vi "Marvin.vi"() -> ()   [LabVIEW 2017]
uses:
  Marvin ATP Remake 1.5.18/PCAN_Driver/ControlCAN.llb/CAN Channel.ctl
  Marvin ATP Remake 6.5.18 - Copy/PCAN_Driver/ControlCAN.llb/DevType.ctl
  Marvin ATP Remake 30.5.18/PCAN_Driver/ControlCAN.llb/VCI_INIT_CONFIG.ctl
  Marvin ATP Remake 30.5.18/PCAN_Driver/ControlCAN.llb/InitFlag.ctl
  Marvin ATP Remake 6.5.18/PCAN_Driver/ControlCAN.llb/Fliter.ctl
  Marvin ATP Remake 6.5.18/PCAN_Driver/ControlCAN.llb/Mode.ctl
  <vilib>/Utility/miscctls.llb/LVMinMaxIncTypeDef.ctl
  PCAN_Driver/ControlCAN.llb/VCI_CAN_OBJ.ctl
  Marvin ATP Remake 30.5.18/PCAN_Driver/ControlCAN.lvlib
panel:
  in  "Graph Plot":bool
  in  "Get":bool
  in  "Set":bool
  out "Array 2":dbl[](array[numeric])
  in  "Clear Data Array":bool
  in  "PlayPause Data Array":bool
  out "CAN Data":cluster{"Frame Data":u64, "Frame ID":u32}[](array[cluster]) {"Frame ID" format="%.0x"; "Frame Data" format="%016x"}
  out "Waveform Chart":dbl(graph)
  in  "Help Button":bool
  in  "Clear Monitor":bool
  out "Array":u64[][](array[numeric]) format="%016x"
  out "Ambient Over temp":bool
  out "Ambient Sensor temp":bool
  out "Ambient Temperature":dbl
  in  "Motor Over Temp":bool
  in  "Speed control":bool
  out "Unit Adress":string
  in  "Serial Send":bool
  in  "Index":u16(ring) items=["1"=1, "2"=2, "3"=3]
  out "read buffer":string
  in  "SetGet":enum16{"Get", "Set"}(ring)
  in  "Function":T1(ring)
  in  "Value":dbl
  in  "Value 1/2":enum16{"1", "2"}(ring)
  out "Msg Count":u32
  in  "Param to Set":u16(ring) items=["EBAY 5F"=95, "AHU 3F"=63, "AHU 2F"=47]
  out "UUT":u8
  out "Horizontal Progress Bar":i32(slide) min=0 max=48 scale=0.0..50.0
  in  "Set Param.":bool
  in  "Serial Monitor":bool caption="Graph Button"
  in  "Serial Com":bool
  in  "VISA resource name":refnum<visa-resource-name>="COM6"
  out "Serial Status":bool
  in  "Graph Button":bool
  in  "Refresh Button":bool
  out "Data Send":u64 format="%016x"
  in  "Motor Speed RPM":u16
  out "Under voltage/Over voltage":bool
  out "Speed error":bool
  out "Derated drive temp":bool
  out "Motor Over temperature":bool
  out "Commutation err":bool
  out "Motor Sensor temp Fauilre":bool
  out "Drive Over temperature":bool
  out "Drive Sensor temp Failure":bool
  out "Motor Phase Current RMS":dbl
  out "ECS State":u16
  out "Motor Speed RPM":dbl
  out "Motor Stator Temp.":dbl
  out "Power transistor Heat sink Temp.":dbl
  out "Phase Current":dbl
  out "DC Voltage":dbl
  in  "Can Send":bool
  in  "Stop":bool
  out "Config_CANAT":T8 {"DevType" items=["USB-CAN"=3, "USB-CAN2"=4]; "CanIndex" items=["通道1", "通道2"]; "VCI_INIT_CONFIG"."Fliter" items=["接收所有类型"=3, "只接收标准帧"=4, "只接收扩展帧"=7]; "VCI_INIT_CONFIG"."Mode" items=["正常工作", "自测模式（环回）", "仅侦听模式"]; "VCI_INIT_CONFIG"."InitFlag" items=["使用Flash参数", "使用界面设置参数"]}
  in  "Channel 2":T3 caption="Channel" items=["Channel 1", "Channel 2"]
  out "CAN Status":bool
  out "Driver Version":string
  out "Hall Sensor Fault":bool
  out "Motor Phase Current":dbl
  in  "Motor Phase Current":u16
  # "ver 0.0.b"
  # "Redler"
  # "REDLER TECHNOLOGIES LTD"
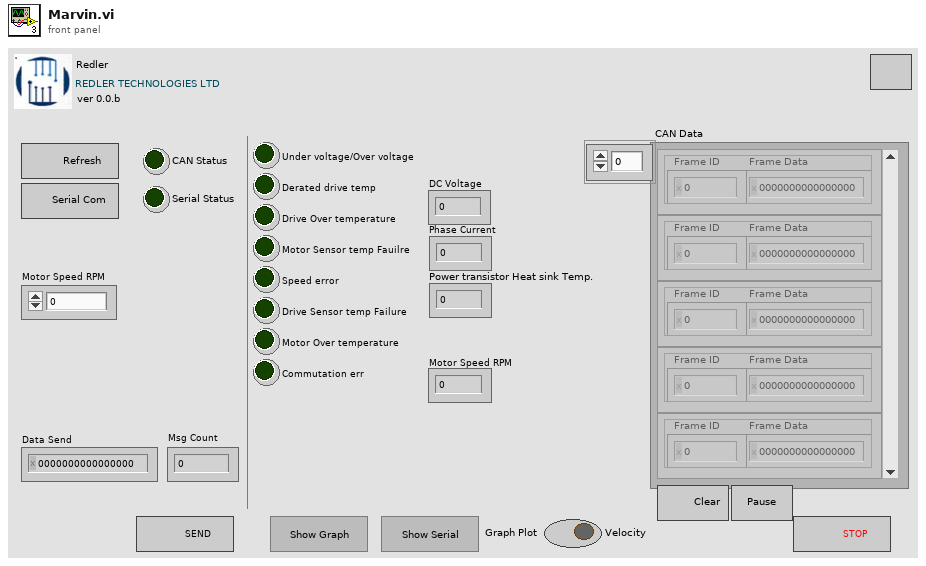
[diagram p1: front panel]
types:
  T1 = enum16{"Enable Conf. EP=1", "Serial Number", "Temperature", "Unit Adress", "Calibration", "Velocity", "Version"}
  T2 = typedef "ControlCAN.lvlib/DevType.ctl" = u32
  T3 = typedef "ControlCAN.lvlib/CAN Channel.ctl" = u32
  T4 = typedef "ControlCAN.lvlib/VCI_INIT_CONFIG.ctl" = cluster{"AccCode":u32, "AccMask":u32, "InitFlag":T5, "Fliter":T6, "Timing0":u8, "Timing1":u8, "Mode":T7}
  T5 = typedef "ControlCAN.lvlib/InitFlag.ctl" = u32
  T6 = typedef "ControlCAN.lvlib/Fliter.ctl" = u8
  T7 = typedef "ControlCAN.lvlib/Mode.ctl" = u8
  T8 = cluster{"DevType":T2, "DevIndex":u32, "CanIndex":T3, "VCI_INIT_CONFIG":T4}
  T9 = cluster{"ID":u32, "MSGTYPE":u8, "LEN":u8, "aDATA":u8[]}[]
  T10 = cluster{"ID":u32, "MSGTYPE":u8, "LEN":u8, "aDATA":u8[]}
  T11 = enum8{"Enabled", "Disabled", "Disabled and Grayed Out"}
  T12 = typedef "LVMinMaxIncTypeDef.ctl" = cluster{"Minimum":dbl, "Maximum":dbl, "Increment":dbl}
  T13 = enum32{"Invalid", "Standard", "Closed", "Hidden", "Minimized", "Maximized"}
  T14 = typedef "ControlCAN.lvlib/VCI_CAN_OBJ.ctl" = cluster{"ID":u32, "TimeStamp":u32, "TimeFlag":u8, "SendType":u8, "RemoteFlag":u8, "ExternFlag":u8, "DataLen":u8, "Data":u8[], "Reserved":u8[]}
  T15 = cluster{"Type":enum16{"接收", "发送"}, "Channel":T3, "Time":timestamp, "VCI_CAN_OBJ":T14}[]
  T16 = cluster{"Type":enum16{"接收", "发送"}, "Channel":T3, "Time":timestamp, "VCI_CAN_OBJ":T14}
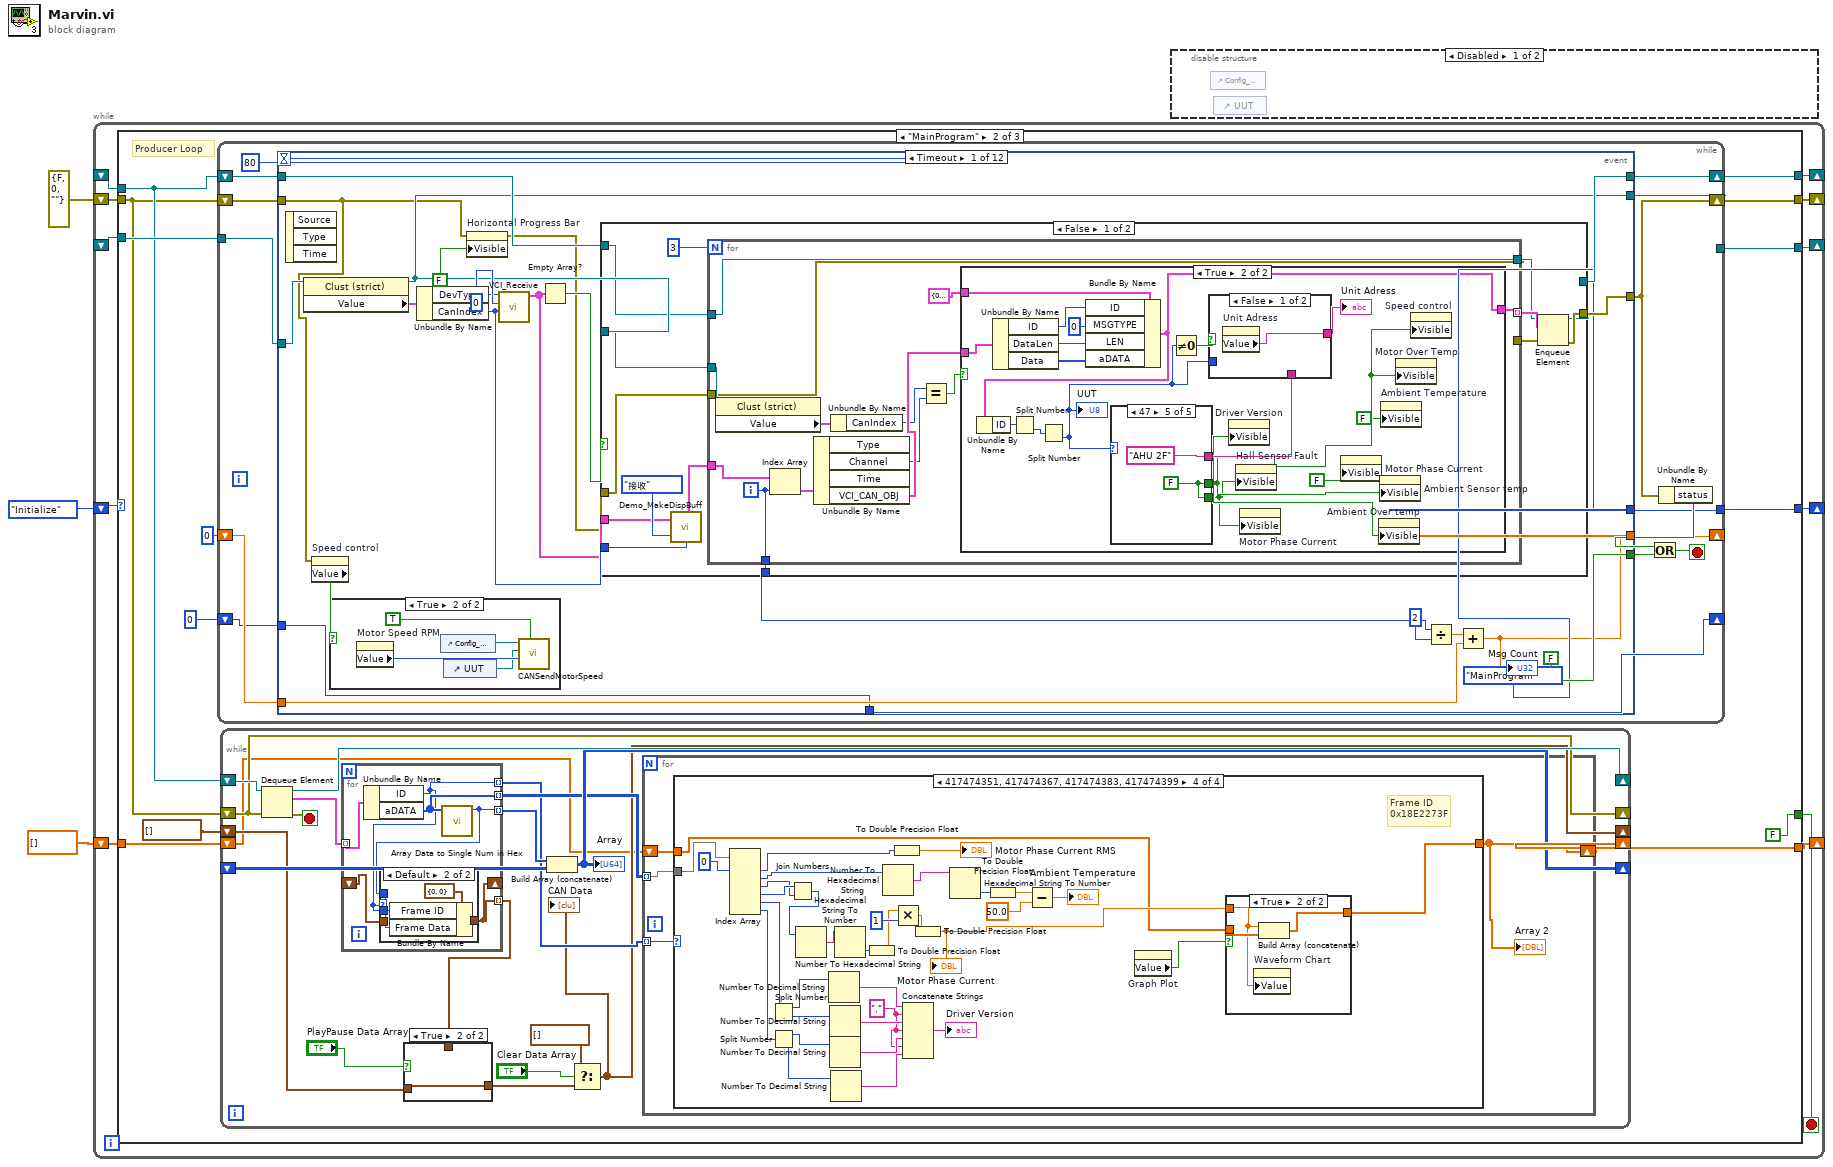
[diagram p0: block diagram]
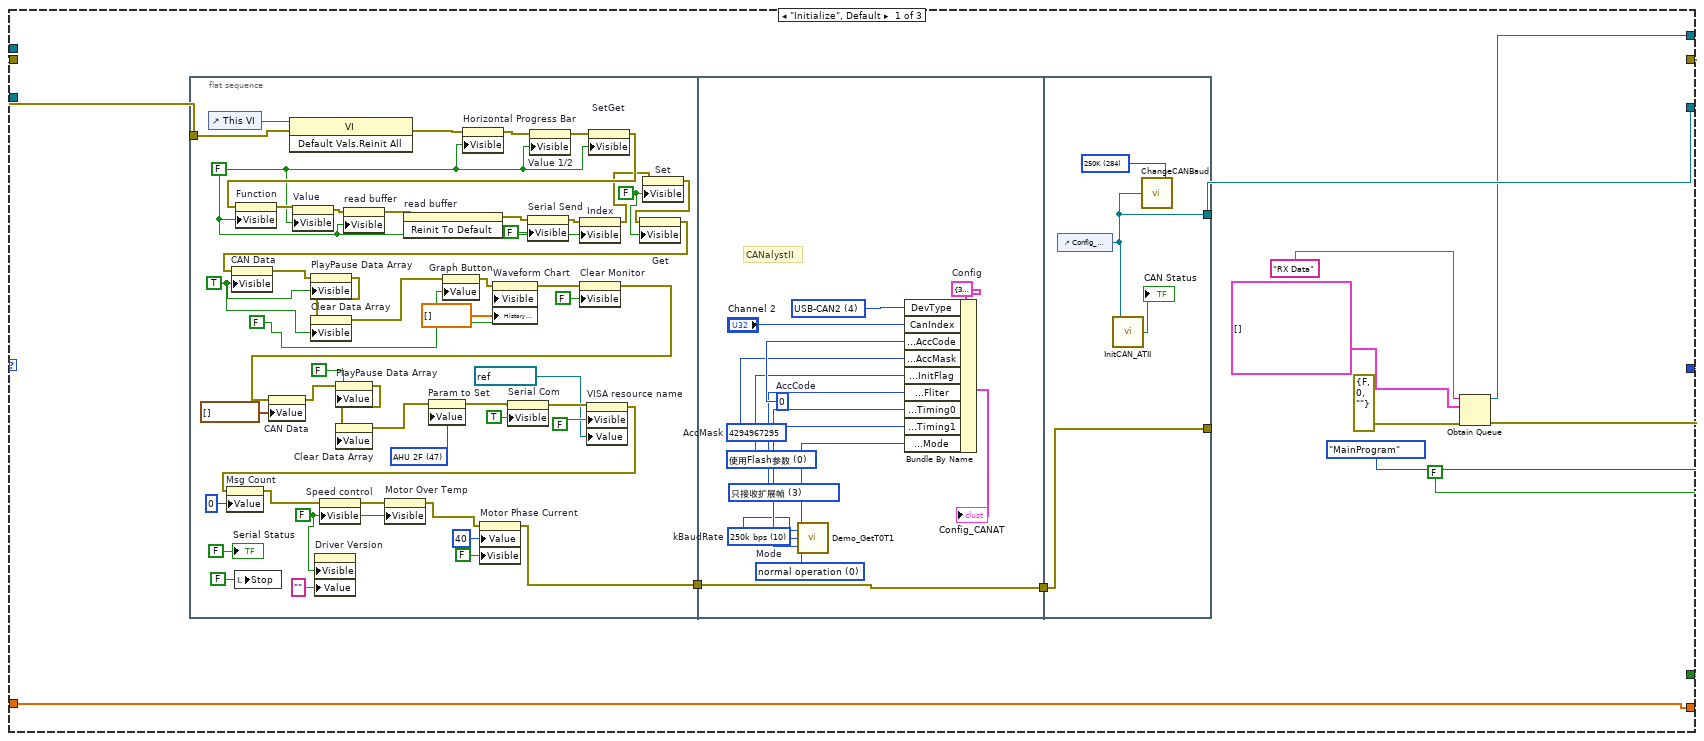
[diagram p3: hidden frame]
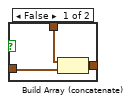
[diagram p4: hidden frame]
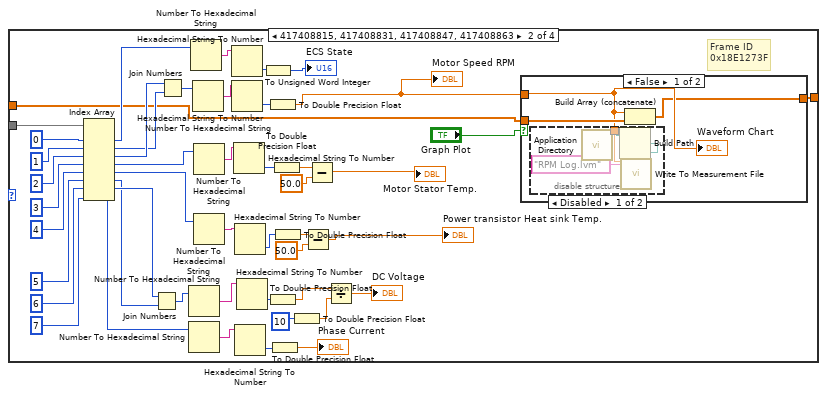
[diagram p6: hidden frame]
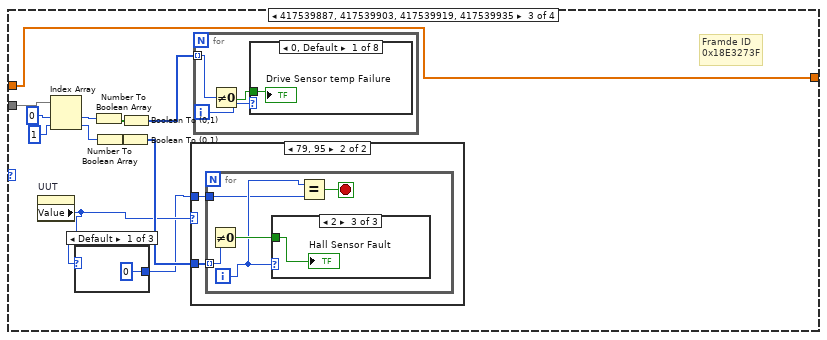
[diagram p9: hidden frame]
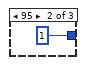
[diagram p10: hidden frame]
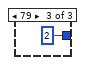
[diagram p11: hidden frame]
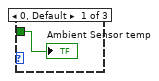
[diagram p13: hidden frame]
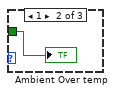
[diagram p14: hidden frame]
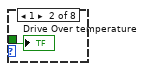
[diagram p15: hidden frame]
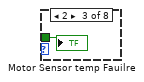
[diagram p16: hidden frame]
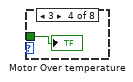
[diagram p17: hidden frame]
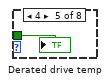
[diagram p18: hidden frame]
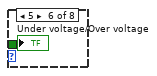
[diagram p19: hidden frame]
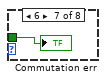
[diagram p20: hidden frame]
diagram:
  n1 = while {
    shift-right: [w9] -> _
    shift-left: enum16{"Stop", "MainProgram", "Initialize"}."Initialize" -> [w14]
    shift-right: [w13] -> _
    shift-left: _ -> [w12]
    shift-right: [w11] -> _
    shift-left: _ -> [w8]
    shift-right: [w10] -> _
    shift-left: errorcluster {"status"=FALSE, "code"=0, "source"=""} ("error out") -> [w7]
    shift-right: [w4] -> _
    shift-left: dbl[] [] -> [w5]
    stop <- w6 stop-if-true
    n2 = case shown="\"MainProgram\"" w14 {
      tunnel: [w26 w103 w1077] -> w13
      tunnel: w12 -> [_ w106 w1077]
      tunnel: [w22 w105 w1078] -> w11
      tunnel: [w21 w104 w1079] -> w10
      tunnel: [enum16{"Stop", "MainProgram", "Initialize"}."MainProgram" w102 enum16{"Stop", "MainProgram", "Initialize"}."Stop"] -> w9
      tunnel: w8 -> [_ w101 w1078]
      tunnel: w7 -> [w19 w100 w1080]
      tunnel: [FALSE ("Stop") FALSE ("Stop") w1076] -> w6
      tunnel: w5 -> [w15 w97 w1074]
      tunnel: [w15 w96 w1074] -> w4
      frame "Initialize", Default {
        n3 = flat-sequence {
          tunnel: w19 -> [w58]
          tunnel: [w34] -> w17
          tunnel: [w77] -> w18
          tunnel: w17 -> [w77]
          tunnel: [w91] -> w26
          tunnel: w18 -> [w90]
          tunnel: [w90] -> _
          frame #0 {
            w31 = FALSE ("Visible")
            w43 = FALSE ("PlayPause Data Array")
            w37 = FALSE ("Visible")
            w68 = u16 47 items=["EBAY 5F"=95, "AHU 3F"=63, "AHU 2F"=47] ("Param to Set")
            w38 = TRUE ("Visible")
            w52 = FALSE ("Visible")
            w42 = FALSE ("Graph Button")
            n4 = control-ref of="This VI"() -> (w76:refnum<vi>)
            n5 = local write "Stop"(FALSE ("Stop")) -> ()
            n6 = invoke class="VI" method="Default Vals.Reinit All"(reference=w76, error in=w58) -> (error out=w57:errorcluster)  [unwired: 1 in, 2 out]
            n7 = property on="Driver Version" class="Str"("Visible"=w37, "Value"="" ("Driver Version")) -> ()  [unwired: 2 in, 2 out]
            n8 = property on="Horizontal Progress Bar" class="Slide (strict)"(error in=w57, "Visible"=w52) -> (error out=w66:errorcluster)  [unwired: 1 in, 1 out]
            n9 = property on="Value 1/2" class="Enum (strict)"(error in=w66, "Visible"=w52) -> (error out=w65:errorcluster)  [unwired: 1 in, 1 out]
            n10 = property on="SetGet" class="Enum (strict)"(error in=w65, "Visible"=w52) -> (error out=w64:errorcluster)  [unwired: 1 in, 1 out]
            n11 = property on="Function" class="Enum (strict)"(error in=w64, "Visible"=w52) -> (error out=w63:errorcluster)  [unwired: 1 in, 1 out]
            n12 = property on="Value" class="DigNum (strict)"(error in=w63, "Visible"=w52) -> (error out=w62:errorcluster)  [unwired: 1 in, 1 out]
            n13 = property on="read buffer" class="Str"(error in=w62, "Visible"=w52) -> (error out=w54:errorcluster)  [unwired: 1 in, 1 out]
            n14 = invoke on="read buffer" class="Str" method="Reinit To Default"(error in=w54) -> (error out=w53:errorcluster)  [unwired: 2 in, 2 out]
            n15 = property on="Serial Send" class="Bool (strict)"(error in=w53, "Visible"=FALSE) -> (error out=w61:errorcluster)  [unwired: 1 in, 1 out]
            n16 = property on="Index" class="Ring (strict)"(error in=w61, "Visible"=w52) -> (error out=w29:errorcluster)  [unwired: 1 in, 1 out]
            n17 = property on="Set" class="Bool (strict)"(error in=w29, "Visible"=w31) -> (error out=w30:errorcluster)  [unwired: 1 in, 1 out]
            n18 = property on="Get" class="Bool (strict)"(error in=w30, "Visible"=w31) -> (error out=w28:errorcluster)  [unwired: 1 in, 1 out]
            n19 = property on="CAN Data" class="Arr (strict)"(error in=w28, "Visible"=w38) -> (error out=w41:errorcluster)  [unwired: 1 in, 1 out]
            n20 = property on="PlayPause Data Array" class="Bool (strict)"(error in=w41, "Visible"=w38) -> (error out=w40:errorcluster)  [unwired: 1 in, 1 out]
            n21 = property on="Clear Data Array" class="Bool (strict)"(error in=w40, "Visible"=w38) -> (error out=w39:errorcluster)  [unwired: 1 in, 1 out]
            n22 = property on="Graph Button" class="Bool (strict)"(error in=w39, "Value"=w42) -> (error out=w50:errorcluster)  [unwired: 1 in, 1 out]
            n23 = property on="Waveform Chart" class="WFChart (strict)"(error in=w50, "Visible"=w42, "History Data"=dbl[] [] ("Waveform Chart")) -> (error out=w49:errorcluster)  [unwired: 1 in, 1 out]
            n24 = property on="Clear Monitor" class="Bool"(error in=w49, "Visible"=FALSE) -> (error out=w48:errorcluster)  [unwired: 1 in, 1 out]
            n25 = property on="CAN Data" class="Arr (strict)"(error in=w48, "Value"=cluster{"Frame Data":u64, "Frame ID":u32}[] [] ("CAN Data")) -> (error out=w46:errorcluster)  [unwired: 1 in, 1 out]
            n26 = property on="PlayPause Data Array" class="Bool (strict)"(error in=w46, "Value"=w43) -> (error out=w45:errorcluster)  [unwired: 1 in, 1 out]
            n27 = property on="Clear Data Array" class="Bool (strict)"(error in=w45, "Value"=w43) -> (error out=w44:errorcluster)  [unwired: 1 in, 1 out]
            n28 = property on="Param to Set" class="Ring (strict)"(error in=w44, "Value"=w68) -> (error out=w60:errorcluster)  [unwired: 1 in, 1 out]
            n29 = property on="Serial Com" class="Bool"(error in=w60, "Visible"=TRUE) -> (error out=w73:errorcluster)  [unwired: 1 in, 1 out]
            n30 = property on="VISA resource name" class="VISAName"(error in=w73, "Visible"=FALSE, "Value"=refnum<visa-resource-name> "COM1" ("VISA resource name")) -> (error out=w59:errorcluster)  [unwired: 1 in, 1 out]
            n31 = property on="Msg Count" class="DigNum (strict)"(error in=w59, "Value"=u32 0 ("Msg Count")) -> (error out=w56:errorcluster)  [unwired: 1 in, 1 out]
            n32 = property on="Speed control" class="Bool (strict)"(error in=w56, "Visible"=w37) -> (error out=w55:errorcluster)  [unwired: 1 in, 1 out]
            n33 = property on="Motor Over Temp" class="Bool (strict)"(error in=w55, "Visible"=w37) -> (error out=w35:errorcluster)  [unwired: 1 in, 1 out]
            n34 = property on="Motor Phase Current" class="DigNum (strict)"(error in=w35, "Value"=u16 40 ("Motor Phase Current"), "Visible"=FALSE) -> (error out=w34:errorcluster)  [unwired: 1 in, 1 out]
            "Serial Status" <- FALSE ("Serial Status")
          }
          frame #1 {
            w81 = u32 4294967295  # AccMask
            w80 = T5 0 items=["使用Flash参数", "使用界面设置参数"] ("InitFlag")
            w78 = T7 0 items=["normal operation", "Listen-only mode", "test mode"]  # Mode
            w79 = T6 3 items=["接收所有类型"=1, "只接收标准帧"=2, "只接收扩展帧"=3] ("Fliter")
            w85 = u8 10 items=["5k bps"=1, "10k bps"=2, "20k bps"=3, "40k bps"=4, "50k bps"=5, "80k bps"=6, "100k bps"=7, "125k bps"=8, "200k bps"=9, "250k bps"=10, "400k bps"=11, "500k bps"=12, "666k bps"=13, "800k bps"=14, "1000k bps"=15, "33.33k bps"=16, "66.66k bps"=17, "83.33k bps"=18]  # kBaudRate
            w82 = u32 0  # AccCode
            w83 = T2 4 items=["USB-CAN"=3, "USB-CAN2"=4] ("DevType")
            w84 = T8 {"DevType"=3, "DevIndex"=0, "CanIndex"=0, "VCI_INIT_CONFIG"={"AccCode"=0, "AccMask"=0, "InitFlag"=1, "Fliter"=7, "Timing0"=0, "Timing1"=0, "Mode"=0}}  # Config
            # "CANalystII"
            n35 = call "Demo_GetT0T1.vi"("kBaudRate"=w85) -> ("Timing0"=w87:u8, "Timing1"=w88:u8)
            n36 = Bundle By Name(cluster=w84, "DevType"=w83, "CanIndex"="Channel 2", "VCI_INIT_CONFIG.AccCode"=w82, "VCI_INIT_CONFIG.AccMask"=w81, "VCI_INIT_CONFIG.InitFlag"=w80, "VCI_INIT_CONFIG.Fliter"=w79, "VCI_INIT_CONFIG.Timing0"=w87, "VCI_INIT_CONFIG.Timing1"=w88, "VCI_INIT_CONFIG.Mode"=w78) -> (→"Config_CANAT":T8)
          }
          frame #2 {
            w92 = u16 284 items=["1M"=20, "500K"=28, "250K"=284, "125K"=796, "100K"=17199, "50K"=18223, "20K"=21295, "10K"=26415, "5K"=32639] ("baud in")
            n37 = control-ref of="Config_CANAT"() -> (w91:refnum<vi>)
            n38 = call "InitCAN_ATII.vi"("Config"=w91) -> ("Sts"=→"CAN Status":bool)
            n39 = call "ChangeCANBaud.vi"("baud in"=w92, "reference"=w91) -> ()
          }
        }
        n40 = Obtain Queue(name (unnamed)="RX Data", element data type=T9 [], error in (no error)=errorcluster {"status"=FALSE, "code"=0, "source"=""}) -> (queue out=w22:refnum<queue>, error out=w21:errorcluster)  [unwired: 2 in, 1 out]
      }
      frame "MainProgram" {
        # "Producer Loop"
        n41 = while {
          shift-right: [w283] -> w104
          shift-left: w100 -> [w285]
          shift-right: [w284] -> w105
          shift-left: w101 -> [w286]
          tunnel: w106 -> [w287]
          tunnel: [w280] -> w103
          tunnel: [w279] -> w102
          shift-right: [w277] -> _
          shift-left: 0 -> [w278]
          shift-right: [w275] -> _
          shift-left: 0 -> [w276]
          stop <- w288 stop-if-true
          n42 = event shown="[0] Timeout" {
            selector: _ -> [_ _ _ _ _ _ _ _ _ _ _ _]
            dyn-events: _ -> [_ _ _ _ _ _ _ _ _ _ _ _]
            timeout: 80 ("Numeric") -> [_ _ _ _ _ _ _ _ _ _ _ _]
            tunnel: w287 -> [w309 w389 w410 w497 w779 w877 w900 w999 w1019 w1036 w1051 w1060]
            tunnel: w286 -> [w306 w390 w413 w498 w778 w878 w921 w1000 w1018 w1037 w1048 w1058]
            tunnel: w285 -> [w291 w388 w408 w474 w771 w870 w920 w980 w1014 w1029 w1047 w1059]
            tunnel: [w304 w390 w413 w498 w778 w878 w921 w1000 w1018 w1037 w1046 w1058] -> w284
            tunnel: [w303 w383 w409 w490 w767 w867 w920 w987 w1011 w1027 w1044 w1057] -> w283
            tunnel: [FALSE ("Stop") FALSE ("Stop") FALSE ("Stop") FALSE ("Stop") FALSE ("Stop") FALSE ("Stop") FALSE ("Stop") FALSE ("Stop") FALSE ("Stop") FALSE ("Stop") TRUE ("Stop") w1053] -> w281
            tunnel: [w302 w389 w410 w497 w779 w877 w900 w999 w1019 w1036 w1051 w1060] -> w280
            tunnel: [enum16{"Stop", "MainProgram", "Initialize"}."MainProgram" enum16{"Stop", "MainProgram", "Initialize"}."MainProgram" enum16{"Stop", "MainProgram", "Initialize"}."MainProgram" enum16{"Stop", "MainProgram", "Initialize"}."MainProgram" enum16{"Stop", "MainProgram", "Initialize"}."MainProgram" enum16{"Stop", "MainProgram", "Initialize"}."MainProgram" enum16{"Stop", "MainProgram", "Initialize"}."MainProgram" enum16{"Stop", "MainProgram", "Initialize"}."MainProgram" enum16{"Stop", "MainProgram", "Initialize"}."MainProgram" enum16{"Stop", "MainProgram", "Initialize"}."MainProgram" enum16{"Stop", "MainProgram", "Initialize"}."Stop" w1052] -> w279
            tunnel: w278 -> [w298 w393 w406 w486 w769 w881 w886 w995 w1010 w1025 w1043 w1056]
            tunnel: [w297 w393 w406 w486 w769 w881 w886 w995 w1010 w1025 w1043 w1056] -> w277
            tunnel: w276 -> [w290 _ _ _ _ _ _ _ _ _ _ _]
            tunnel: [w290 _ _ _ _ _ _ _ _ _ _ _] -> w275
            event Timeout {
              n43 = event-data() -> ()  [unwired: 1 in, 3 out]
              n44 = property class="Clust (strict)"(reference=w309) -> (reference out=w302:refnum<vi>, "Value"=w310:T8)  [unwired: 1 in, 1 out]
              n45 = property on="Speed control" class="Bool (strict)"(error in=w291) -> ("Value"=w292:bool)  [unwired: 1 in, 2 out]
              n46 = case shown="True" w292 {
                frame False {
                }
                frame True {
                  n47 = property on="Motor Speed RPM" class="DigNum (strict)"() -> ("Value"=w316:u16)  [unwired: 2 in, 2 out]
                  n48 = control-ref of="Config_CANAT"() -> (w315:refnum<vi>)
                  n49 = control-ref of="UUT"() -> (w314:refnum<vi>)
                  n50 = call "CANSendMotorSpeed.vi"("Remote"=TRUE, "Motor Speed RPM"=w316, "UUT"=w314, "CAN Cluster in"=w315) -> ()  [unwired: 7 in, 1 out]
                }
              }
              n51 = Unbundle By Name(w310) -> ("DevType"=w311:T2, "CanIndex"=w307:T3)
              n52 = property on="Horizontal Progress Bar" class="Slide (strict)"(error in=w291, "Visible"=FALSE) -> (error out=w293:errorcluster)  [unwired: 1 in, 1 out]
              n53 = call "VCI_Receive.vi"("CANIndex"=w307, "DevIndex"=u32 0, "DevType"=w311) -> ("Recieve"=w305:T14[])  [unwired: 3 in, 5 out]
              n54 = Empty Array?(array=w305) -> (empty?=w308:bool)
              n55 = case shown="False" w308 {
                tunnel: w307 -> [w328 _]
                tunnel: w302 -> [w326 _]
                tunnel: w306 -> [w325 w382]
                tunnel: w293 -> [w324 w381]
                tunnel: w305 -> [w329 _]
                tunnel: [w319 w381] -> w303
                tunnel: [w318 w382] -> w304
                tunnel: [w317 0] -> w294
                frame False {
                  n56 = call "Demo_MakeDispBuff.vi"("Channel"=w328, "Type"=enum16{"接收", "发送"}."接收", "OBJs"=w329) -> ("Buffer"=w327:T15)
                  n57 = for {
                    N: 3 -> [_]
                    tunnel: w327 -> [w343]
                    tunnel: w326 -> [w342]
                    tunnel: w325 -> [w333]
                    tunnel: w324 -> [w332]
                    tunnel: [w335] -> w322 mode=indexing
                    tunnel: [w333] -> w321
                    tunnel: [w332] -> w320
                    tunnel: [w331] -> w317
                    i -> [w331]
                    n58 = property class="Clust (strict)"(reference=w342) -> ("Value"=w340:T8)  [unwired: 1 in, 2 out]
                    n59 = Index Array(array=w343, index=w331) -> (element=w336:T16)
                    n60 = Unbundle By Name(w336) -> ("Channel"=w338:T3, "VCI_CAN_OBJ"=w341:T14)  [unwired: 2 out]
                    n61 = Unbundle By Name(w340) -> ("CanIndex"=w339:T3)
                    n62 = Equal?(x=w339, y=w338) -> (x = y?=w337:bool)
                    n63 = case shown="True" w337 {
                      tunnel: w341 -> [_ w361]
                      tunnel: [w344 w357] -> w335
                      tunnel: T10 {"ID"=0, "MSGTYPE"=0, "LEN"=0, "aDATA"=[]} ("Msg") -> [w344 w356]
                      frame False {
                      }
                      frame True {
                        n64 = Unbundle By Name(w361) -> ("ID"=w355:u32, "DataLen"=w360:u8, "Data"=w358:u8[])
                        n65 = Bundle By Name(cluster=w356, "ID"=w355, "MSGTYPE"=u8 0, "LEN"=w360, "aDATA"=w358) -> (w357:T10)
                        n66 = Unbundle By Name(w357) -> ("ID"=w353:u32)
                        n67 = Split Number(x=w353) -> (lo(x)=w354:u16)  [unwired: 1 out]
                        n68 = Split Number(x=w354) -> (lo(x)=w351:u8)  [unwired: 1 out]
                        "UUT" <- w351
                        n69 = case shown="47" w351 {
                          tunnel: ["EBAY 5F" "PUMP 4F" w374 "AHU 3F" "AHU 2F"] -> w350
                          tunnel: [TRUE w371 w375 w376 w378] -> w348
                          tunnel: [FALSE w371 w373 w376 w378] -> w347
                          frame 95 {
                          }
                          frame 79 {
                            w371 = TRUE
                          }
                          frame Default {
                            n70 = property on="Hall Sensor Fault" class="Bool (strict)"() -> ("Visible"=w373:bool)  [unwired: 2 in, 2 out]
                            n71 = property on="Speed control" class="Bool (strict)"() -> ("Visible"=w375:bool)  [unwired: 2 in, 2 out]
                            n72 = property on="Unit Adress" class="Str"() -> ("Value"=w374:string)  [unwired: 2 in, 2 out]
                          }
                          frame 63 {
                            w376 = FALSE
                          }
                          frame 47 {
                            w378 = FALSE
                          }
                        }
                        n73 = Not Equal To 0?(x=w351) -> (x != 0?=w352:bool)
                        n74 = case shown="False" w352 {
                          tunnel: w351 -> [_ w367]
                          tunnel: w350 -> [_ w364]
                          tunnel: [w362 w363] -> w349
                          frame False {
                            n75 = property on="Unit Adress" class="Str"() -> ("Value"=w362:string)  [unwired: 2 in, 2 out]
                          }
                          frame True {
                            n76 = Number To Decimal String(number=w367) -> (decimal integer string=w366:string)  [unwired: 1 in]
                            n77 = call <vilib>:"Space Constant.vi"() -> ("String"=w365:string)
                            n78 = Concatenate Strings(w366, w365, w364) -> (w363:string)
                          }
                        }
                        "Unit Adress" <- w349
                        n79 = property on="Driver Version" class="Str"("Visible"=w348) -> ()  [unwired: 2 in, 2 out]
                        n80 = property on="Hall Sensor Fault" class="Bool (strict)"("Visible"=w347) -> ()  [unwired: 2 in, 2 out]
                        n81 = property on="Motor Phase Current" class="DigNum (strict)"("Visible"=w347) -> ()  [unwired: 2 in, 2 out]
                        n82 = property on="Motor Phase Current" class="DigNum (strict)"("Visible"=FALSE) -> ()  [unwired: 2 in, 2 out]
                        n83 = property on="Ambient Over temp" class="Bool (strict)"("Visible"=w348) -> ()  [unwired: 2 in, 2 out]
                        n84 = property on="Ambient Sensor temp" class="Bool (strict)"("Visible"=w348) -> ()  [unwired: 2 in, 2 out]
                        n85 = property on="Ambient Temperature" class="DigNum (strict)"("Visible"=FALSE) -> ()  [unwired: 2 in, 2 out]
                        n86 = property on="Motor Over Temp" class="Bool (strict)"("Visible"=w348) -> ()  [unwired: 2 in, 2 out]
                        n87 = property on="Speed control" class="Bool (strict)"("Visible"=w348) -> ()  [unwired: 2 in, 2 out]
                      }
                    }
                  }
                  n88 = Enqueue Element(queue=w321, element=w322, error in (no error)=w320) -> (queue out=w318:refnum<queue>, error out=w319:errorcluster)  [unwired: 2 out]
                }
                frame True {
                }
              }
              n89 = Divide(x=w294, y=u32 2) -> (x/y=w295:dbl)
              n90 = Add(x=w295, y=w298) -> (x+y=w297:dbl)
              "Msg Count" <- w297
            }
            event "Clear Monitor": Value Change {
              n91 = event-data() -> ()  [unwired: 1 in, 6 out]
              n92 = property on="VISA resource name" class="VISAName"(error in=w388) -> (error out=w387:errorcluster, "Value"=w386:refnum<visa-resource-name>)  [unwired: 1 in, 1 out]
              n93 = disable-structure shown="Enabled" {
                disable-tunnel: w387 -> [w398 w401]
                disable-tunnel: w386 -> [w396 w402]
                disable-tunnel: [w395 ""] -> w385
                disable-tunnel: [w394 w400] -> w384
                frame Disabled {
                  n94 = call "Serial.vi"("error in (no error)"=w398, "Clear Log"=TRUE, "VISA resource name"=w396) -> ("error out"=w394:errorcluster, "read buffer"=w395:string)  [unwired: 7 in]
                }
                frame Enabled {
                  n95 = VISA Flush I/O Buffer(VISA resource name=w402, error in (no error)=w401) -> (error out=w400:errorcluster)  [unwired: 1 in, 1 out]
                }
              }
              n96 = property on="read buffer" class="Str"(error in=w384, "Value"=w385) -> (error out=w383:errorcluster)  [unwired: 1 in, 1 out]
            }
            event "Serial Monitor": Value Change {
              n97 = event-data() -> ()  [unwired: 1 in, 6 out]
              n98 = property on="Serial Status" class="Bool (strict)"(error in=w408) -> (error out=w407:errorcluster, "Value"=w405:bool)  [unwired: 1 in, 1 out]
              n99 = Or(x=FALSE, y=w405) -> (x .or. y?=w404:bool)
              n100 = case shown="True" w404 {
                tunnel: w407 -> [w417 w436]
                tunnel: [w415 w441] -> w409
                frame False {
                  n101 = call "Display Message to User3"("error in (no error)"=w417) -> ("error out"=w416:errorcluster)  [unwired: 9 in, 1 out]
                  n102 = property on="Serial Monitor" class="Bool (strict)"(error in=w416, "Value"=FALSE ("Serial Monitor")) -> (error out=w415:errorcluster)  [unwired: 1 in, 1 out]
                }
                frame True {
                  w424 = FALSE ("Visible")
                  w429 = FALSE ("Visible")
                  w438 = FALSE ("Visible")
                  w439 = u16 1 items=["1"=1, "2"=2, "3"=3] ("Index")
                  n103 = property on="Index" class="Ring (strict)"(error in=w436, "Value"=w439) -> (error out=w435:errorcluster)  [unwired: 1 in, 1 out]
                  n104 = property on="Value 1/2" class="Enum (strict)"(error in=w435, "Visible"=w438) -> (error out=w434:errorcluster)  [unwired: 1 in, 1 out]
                  n105 = property on="Value" class="DigNum (strict)"(error in=w434, "Visible"=w438) -> (error out=w433:errorcluster)  [unwired: 1 in, 1 out]
                  n106 = property on="SetGet" class="Enum (strict)"(error in=w433, "Value"=enum16{"Get", "Set"}."Get" ("SetGet")) -> (error out=w422:errorcluster)  [unwired: 1 in, 1 out]
                  n107 = property on="Set" class="Bool (strict)"(error in=w422, "Visible"=w424) -> (error out=w423:errorcluster)  [unwired: 1 in, 1 out]
                  n108 = property on="Get" class="Bool (strict)"(error in=w423, "Visible"=w424) -> (error out=w421:errorcluster)  [unwired: 1 in, 1 out]
                  n109 = property on="Serial Send" class="Bool (strict)"(error in=w421, "Visible"=w429) -> (error out=w428:errorcluster)  [unwired: 1 in, 1 out]
                  n110 = property on="Clear Monitor" class="Bool"(error in=w428, "Visible"=w429) -> (error out=w427:errorcluster)  [unwired: 1 in, 1 out]
                  n111 = property on="Function" class="Enum (strict)"(error in=w427, "Value"=T1."Serial Number" ("Function")) -> (error out=w432:errorcluster)  [unwired: 1 in, 1 out]
                  n112 = property on="Index" class="Ring (strict)"(error in=w432, "DisabledEnum"=T11."Disabled and Grayed Out" ("Disabled")) -> (error out=w430:errorcluster)  [unwired: 1 in, 1 out]
                  n113 = case shown="True" "Serial Monitor" {
                    selector: "Serial Monitor" -> [w447 w469]
                    tunnel: w430 -> [w446 w465]
                    tunnel: [w448 w466] -> w441
                    tunnel: [w442 TRUE] -> w426
                    tunnel: [FALSE ("Visible") TRUE ("Visible")] -> w419
                    tunnel: [w442 FALSE ("Visible")] -> w418
                    frame False {
                      w442 = FALSE
                      n114 = property on="Graph Button" class="Bool (strict)"(error in=w446) -> (error out=w445:errorcluster, "Value"=w444:bool)  [unwired: 1 in, 1 out]
                      n115 = case shown="True" w444 {
                        tunnel: [w452 w457] -> w449
                        tunnel: w445 -> [w454 w460]
                        tunnel: w447 -> [w455 _]
                        frame False {
                          n116 = property on="Waveform Chart" class="WFChart (strict)"(error in=w454, "Visible"=FALSE) -> (error out=w451:errorcluster)  [unwired: 1 in, 1 out]
                          n117 = Not(x=w455) -> (.not. x?=w450:bool)
                          n118 = property on="PlayPause Data Array" class="Bool (strict)"("Visible"=w450) -> ()  [unwired: 2 in, 2 out]
                          n119 = property on="Clear Data Array" class="Bool (strict)"("Visible"=w450) -> ()  [unwired: 2 in, 2 out]
                          n120 = property on="CAN Data" class="Arr (strict)"(error in=w451, "Visible"=w450) -> (error out=w452:errorcluster)  [unwired: 1 in, 1 out]
                        }
                        frame True {
                          w456 = FALSE ("Visible")
                          n121 = property on="Waveform Chart" class="WFChart (strict)"(error in=w460, "Visible"=TRUE) -> (error out=w458:errorcluster)  [unwired: 1 in, 1 out]
                          n122 = property on="PlayPause Data Array" class="Bool (strict)"("Visible"=w456) -> ()  [unwired: 2 in, 2 out]
                          n123 = property on="Clear Data Array" class="Bool (strict)"("Visible"=w456) -> ()  [unwired: 2 in, 2 out]
                          n124 = property on="CAN Data" class="Arr (strict)"(error in=w458, "Visible"=w456) -> (error out=w457:errorcluster)  [unwired: 1 in, 1 out]
                        }
                      }
                      n125 = property on="Serial Monitor" class="Bool (strict)"(error in=w449, "Value"=w447) -> (error out=w448:errorcluster)  [unwired: 1 in, 1 out]
                    }
                    frame True {
                      n126 = Not(x=w469) -> (.not. x?=w463:bool)
                      n127 = property on="PlayPause Data Array" class="Bool (strict)"("Visible"=w463) -> ()  [unwired: 2 in, 2 out]
                      n128 = property on="CAN Data" class="Arr (strict)"(error in=w465, "Visible"=w463) -> (error out=w464:errorcluster)  [unwired: 1 in, 1 out]
                      n129 = property on="Clear Data Array" class="Bool (strict)"("Visible"=w463) -> ()  [unwired: 2 in, 2 out]
                      n130 = property on="Serial Monitor" class="Bool (strict)"(error in=w464, "Value"=w469) -> (error out=w468:errorcluster)  [unwired: 1 in, 1 out]
                      n131 = property on="Graph Button" class="Bool (strict)"(error in=w468, "Value"=w463) -> (error out=w467:errorcluster)  [unwired: 1 in, 1 out]
                      n132 = property on="Waveform Chart" class="WFChart (strict)"(error in=w467, "Visible"=w463) -> (error out=w466:errorcluster)  [unwired: 1 in, 1 out]
                    }
                  }
                  n133 = property on="Index" class="Ring (strict)"("Visible"=w426) -> ()  [unwired: 2 in, 2 out]
                  n134 = property on="SetGet" class="Enum (strict)"("Visible"=w418) -> ()  [unwired: 2 in, 2 out]
                  n135 = property on="Clear Monitor" class="Bool"("Visible"=w426) -> ()  [unwired: 2 in, 2 out]
                  n136 = property on="Function" class="Enum (strict)"("Visible"=w426) -> ()  [unwired: 2 in, 2 out]
                  n137 = property on="Serial Send" class="Bool (strict)"("Visible"=w418) -> ()  [unwired: 2 in, 2 out]
                  n138 = property on="read buffer" class="Str"("Visible"=w426) -> ()  [unwired: 2 in, 2 out]
                  n139 = property on="Set" class="Bool (strict)"("Visible"=w419) -> (error out=w420:errorcluster)  [unwired: 2 in, 1 out]
                  n140 = property on="Get" class="Bool (strict)"(error in=w420, "Visible"=w419) -> ()  [unwired: 1 in, 2 out]
                }
              }
            }
            event "Serial Send", "SetGet", "Set", "Get", "Function": Value Change; "Function": Mouse Move {
              n141 = event-data() -> ("CtlRef"=w485:refnum<vi>)  [unwired: 1 in, 3 out]
              n142 = property class="Ctl"(reference=w485) -> ("Label.Text"=w484:string)  [unwired: 1 in, 2 out]
              n143 = disable-structure shown="Enabled" {
                disable-tunnel: "Function" -> [w504 _]
                disable-tunnel: w474 -> [w503 w531]
                disable-tunnel: [w502 w531] -> w471
                frame Disabled {
                  n144 = case shown="\"Serial Number\"" w504 {
                    tunnel: w503 -> [w506 w511 w518 w520 w523 w527 w529 w530]
                    tunnel: [w505 w513 w517 w522 w525 w526 w529 w530] -> w502
                    frame "Serial Number" {
                      n145 = property on="Index" class="Ring (strict)"(error in=w506, "DisabledEnum"=T11."Disabled and Grayed Out" ("Disabled")) -> (error out=w505:errorcluster)  [unwired: 1 in, 1 out]
                    }
                    frame "Temperature" {
                      n146 = property on="UUT" class="DigNum (strict)"() -> ("Value"=w508:u8)  [unwired: 2 in, 2 out]
                      n147 = case shown="95" w508 {
                        tunnel: [i32[] [2] ("Disabled Items []") i32[] [3] ("Disabled Items []")] -> w509
                        frame 47, 63, Default {
                        }
                        frame 95 {
                        }
                      }
                      n148 = property on="Index" class="Ring (strict)"(error in=w511, "DisabledEnum"=T11."Enabled" ("Disabled"), "Visible"=TRUE, "Disabled Items []"=w509) -> (error out=w513:errorcluster)  [unwired: 1 in, 1 out]
                    }
                    frame "Unit Adress" {
                      n149 = property on="Index" class="Ring (strict)"(error in=w518, "DisabledEnum"=T11."Enabled" ("Disabled"), "Visible"=TRUE) -> (error out=w517:errorcluster)  [unwired: 1 in, 1 out]
                    }
                    frame "Calibration" {
                      n150 = property on="Index" class="Ring (strict)"(error in=w520, "DisabledEnum"=T11."Disabled and Grayed Out" ("Disabled")) -> (error out=w522:errorcluster)  [unwired: 1 in, 1 out]
                    }
                    frame "Velocity" {
                      n151 = property on="Index" class="Ring (strict)"(error in=w523, "DisabledEnum"=T11."Disabled and Grayed Out" ("Disabled")) -> (error out=w525:errorcluster)  [unwired: 1 in, 1 out]
                    }
                    frame "Version" {
                      n152 = property on="Index" class="Ring (strict)"(error in=w527, "DisabledEnum"=T11."Disabled and Grayed Out" ("Disabled")) -> (error out=w526:errorcluster)  [unwired: 1 in, 1 out]
                    }
                    frame "Enable Conf. EP=1" {
                    }
                    frame Default {
                    }
                  }
                }
                frame Enabled {
                }
              }
              n153 = case shown="\"Temperature\"" "Function" {
                tunnel: w471 -> [w535 w539 w543 w547 w551 w555 w557 w559]
                tunnel: [FALSE TRUE TRUE FALSE FALSE FALSE w556 w558] -> w477
                tunnel: [TRUE FALSE TRUE FALSE TRUE FALSE w556 w558] -> w478
                tunnel: [FALSE FALSE FALSE TRUE FALSE FALSE w556 w558] -> w473
                tunnel: [w535 w539 w543 w547 w551 w555 w557 w559] -> w480
                frame "Serial Number" {
                }
                frame "Temperature" {
                }
                frame "Unit Adress" {
                }
                frame "Calibration" {
                }
                frame "Velocity" {
                }
                frame "Version" {
                }
                frame "Enable Conf. EP=1" {
                  w556 = FALSE
                }
                frame Default {
                  w558 = FALSE
                }
              }
              n154 = property on="Index" class="Ring (strict)"(error in=w480, "Visible"=w477) -> (error out=w476:errorcluster)  [unwired: 1 in, 1 out]
              n155 = property on="Value" class="DigNum (strict)"(error in=w476, "Visible"=w478) -> (error out=w479:errorcluster)  [unwired: 1 in, 1 out]
              n156 = property on="Value 1/2" class="Enum (strict)"(error in=w479, "Visible"=w473) -> (error out=w472:errorcluster)  [unwired: 1 in, 1 out]
              n157 = property on="VISA resource name" class="VISAName"() -> ("Value"=w499:refnum<visa-resource-name>)  [unwired: 2 in, 2 out]
              n158 = property on="read buffer" class="Str"(error in=w471) -> (error out=w492:errorcluster, "Text.Scroll Position"=w489:u32)  [unwired: 1 in, 1 out]
              n159 = Or(x="Set", y="Get") -> (x .or. y?=w483:bool)
              n160 = case shown="\"Get\"" w484 {
                tunnel: "Function" -> [w563 _ w678]
                tunnel: w499 -> [w567 _ w688]
                tunnel: w492 -> [w565 w675 w676]
                tunnel: "Value" -> [_ _ w687]
                tunnel: "Value 1/2" -> [_ _ w685]
                tunnel: "Index" -> [w564 _ w682]
                tunnel: [w566 w675 w680] -> w491
                tunnel: [w561 w674 w679] -> w496
                tunnel: w483 -> [w560 _ w677]
                tunnel: w472 -> [_ _ _]
                frame "Get" {
                  n161 = disable-structure shown="Enabled" {
                    disable-tunnel: w565 -> [w570 _]
                    disable-tunnel: [w568 _] -> w562
                    frame Disabled {
                      w571 = TRUE ("Visible")
                      n162 = property on="Value" class="DigNum (strict)"(error in=w570, "Visible"=w571) -> (error out=w569:errorcluster)  [unwired: 1 in, 1 out]
                      n163 = property on="Value 1/2" class="Enum (strict)"(error in=w569, "Visible"=w571) -> (error out=w568:errorcluster)  [unwired: 1 in, 1 out]
                    }
                    frame Enabled {
                    }
                  }
                  n164 = case shown="True" w560 {
                    tunnel: w567 -> [_ w583]
                    tunnel: [w572 w579] -> w566
                    tunnel: w564 -> [_ w582]
                    tunnel: w563 -> [_ w581]
                    tunnel: w562 -> [w572 w580]
                    tunnel: [w573 w577] -> w561
                    frame False {
                      n165 = property on="read buffer" class="Str"() -> ("Value"=w573:string)  [unwired: 2 in, 2 out]
                    }
                    frame True {
                      w575 = FALSE ("Serial Send")
                      n166 = case shown="\"Serial Number\"" w581 {
                        tunnel: w583 -> [w587 w607 w626 w639 w649 w663 _]
                        tunnel: w580 -> [w586 w599 w617 w635 w648 w662 w672]
                        tunnel: [w590 w608 w627 w640 w653 w664 w672] -> w579
                        tunnel: [w589 w609 w625 w641 w654 w660 "Cannot perform operation.\n" ("read buffer")] -> w578
                        tunnel: w582 -> [_ w602 w618 _ _ _ _]
                        frame "Serial Number" {
                          n167 = disable-structure shown="Enabled" {
                            disable-tunnel: w586 -> [w594 w596]
                            disable-tunnel: [w593 w596] -> w585
                            frame Disabled {
                              n168 = property on="Index" class="Ring (strict)"(error in=w594, "DisabledEnum"=T11."Disabled and Grayed Out" ("Disabled")) -> (error out=w593:errorcluster)  [unwired: 1 in, 1 out]
                            }
                            frame Enabled {
                            }
                          }
                          n169 = Concatenate Strings("SN" ("string"), "\r\n" ("write buffer")) -> (w588:string)
                          n170 = call "Serial.vi"("error in (no error)"=w585, "Clear Log"=FALSE, "write buffer"=w588, "VISA resource name"=w587) -> ("error out"=w590:errorcluster, "read buffer"=w589:string)  [unwired: 6 in]
                        }
                        frame "Temperature" {
                          n171 = disable-structure shown="Enabled" {
                            disable-tunnel: w599 -> [w612 w614]
                            disable-tunnel: [w611 w614] -> w598
                            frame Disabled {
                              n172 = property on="Index" class="Ring (strict)"(error in=w612, "DisabledEnum"=T11."Enabled" ("Disabled"), "Visible"=TRUE) -> (error out=w611:errorcluster)  [unwired: 1 in, 1 out]
                            }
                            frame Enabled {
                            }
                          }
                          n173 = Number To Decimal String(number=w602) -> (decimal integer string=w601:string)  [unwired: 1 in]
                          n174 = Concatenate Strings("TA" ("string"), "[", w601, "]", "\r\n" ("write buffer")) -> (w603:string)
                          n175 = call "Serial.vi"("error in (no error)"=w598, "Clear Log"=FALSE, "write buffer"=w603, "VISA resource name"=w607) -> ("error out"=w608:errorcluster, "read buffer"=w609:string)  [unwired: 6 in]
                        }
                        frame "Unit Adress" {
                          n176 = disable-structure shown="Enabled" {
                            disable-tunnel: w617 -> [w630 w632]
                            disable-tunnel: [w629 w632] -> w616
                            frame Disabled {
                              n177 = property on="Index" class="Ring (strict)"(error in=w630, "DisabledEnum"=T11."Enabled" ("Disabled"), "Visible"=TRUE) -> (error out=w629:errorcluster)  [unwired: 1 in, 1 out]
                            }
                            frame Enabled {
                            }
                          }
                          n178 = Number To Decimal String(number=w618) -> (decimal integer string=w624:string)  [unwired: 1 in]
                          n179 = Concatenate Strings("UA" ("string"), "[", w624, "]", "\r\n" ("write buffer")) -> (w619:string)
                          n180 = call "Serial.vi"("error in (no error)"=w616, "Clear Log"=FALSE, "write buffer"=w619, "VISA resource name"=w626) -> ("error out"=w627:errorcluster, "read buffer"=w625:string)  [unwired: 6 in]
                        }
                        frame "Calibration" {
                          n181 = disable-structure shown="Enabled" {
                            disable-tunnel: w635 -> [w643 w645]
                            disable-tunnel: [w642 w645] -> w634
                            frame Disabled {
                              n182 = property on="Index" class="Ring (strict)"(error in=w643, "DisabledEnum"=T11."Disabled and Grayed Out" ("Disabled")) -> (error out=w642:errorcluster)  [unwired: 1 in, 1 out]
                            }
                            frame Enabled {
                            }
                          }
                          n183 = Concatenate Strings("CC" ("string"), "\r\n" ("write buffer")) -> (w637:string)
                          n184 = call "Serial.vi"("error in (no error)"=w634, "Clear Log"=FALSE, "write buffer"=w637, "VISA resource name"=w639) -> ("error out"=w640:errorcluster, "read buffer"=w641:string)  [unwired: 6 in]
                        }
                        frame "Velocity" {
                          n185 = disable-structure shown="Enabled" {
                            disable-tunnel: w648 -> [w656 w658]
                            disable-tunnel: [w655 w658] -> w647
                            frame Disabled {
                              n186 = property on="Index" class="Ring (strict)"(error in=w656, "DisabledEnum"=T11."Disabled and Grayed Out" ("Disabled")) -> (error out=w655:errorcluster)  [unwired: 1 in, 1 out]
                            }
                            frame Enabled {
                            }
                          }
                          n187 = Concatenate Strings("VC" ("string"), "\r\n" ("write buffer")) -> (w650:string)
                          n188 = call "Serial.vi"("error in (no error)"=w647, "Clear Log"=FALSE, "write buffer"=w650, "VISA resource name"=w649) -> ("error out"=w653:errorcluster, "read buffer"=w654:string)  [unwired: 6 in]
                        }
                        frame "Version" {
                          n189 = disable-structure shown="Enabled" {
                            disable-tunnel: w662 -> [w669 w671]
                            disable-tunnel: [w668 w671] -> w661
                            frame Disabled {
                              n190 = property on="Index" class="Ring (strict)"(error in=w669, "DisabledEnum"=T11."Disabled and Grayed Out" ("Disabled")) -> (error out=w668:errorcluster)  [unwired: 1 in, 1 out]
                            }
                            frame Enabled {
                            }
                          }
                          n191 = Concatenate Strings("VR" ("string"), "\r\n" ("write buffer")) -> (w665:string)
                          n192 = call "Serial.vi"("error in (no error)"=w661, "Clear Log"=FALSE, "write buffer"=w665, "VISA resource name"=w663) -> ("error out"=w664:errorcluster, "read buffer"=w660:string)  [unwired: 6 in]
                        }
                        frame Default {
                        }
                      }
                      n193 = property on="Serial Send" class="Bool (strict)"(error in=w579, "Value"=w575) -> (error out=w574:errorcluster)  [unwired: 1 in, 1 out]
                      n194 = property on="read buffer" class="Str"() -> ("Value"=w576:string)  [unwired: 2 in, 2 out]
                      n195 = Concatenate Strings(w576, w578) -> (w577:string)
                      n196 = property on="Get" class="Bool (strict)"(error in=w574, "Value"=w575) -> ()  [unwired: 1 in, 2 out]
                    }
                  }
                }
                frame Default {
                  n197 = property on="read buffer" class="Str"() -> ("Value"=w674:string)  [unwired: 2 in, 2 out]
                }
                frame "Set" {
                  n198 = To Unsigned Long Integer(number=w687) -> (unsigned 32bit integer=w683:u32)
                  n199 = Number To Decimal String(number=w682) -> (decimal integer string=w681:string)  [unwired: 1 in]
                  n200 = Number To Decimal String(number=w685) -> (decimal integer string=w684:string)  [unwired: 1 in]
                  n201 = Number To Decimal String(number=w683) -> (decimal integer string=w686:string)  [unwired: 1 in]
                  n202 = case shown="True" w677 {
                    tunnel: w688 -> [_ w705]
                    tunnel: w686 -> [_ w704]
                    tunnel: w684 -> [_ w703]
                    tunnel: w683 -> [_ w702]
                    tunnel: w681 -> [_ w701]
                    tunnel: [w689 w692] -> w680
                    tunnel: [w690 w700] -> w679
                    tunnel: w678 -> [_ w698]
                    tunnel: w676 -> [w689 w697]
                    frame False {
                      n203 = property on="read buffer" class="Str"() -> ("Value"=w690:string)  [unwired: 2 in, 2 out]
                    }
                    frame True {
                      w691 = TRUE ("Value (Signaling)")
                      w694 = FALSE ("Serial Send")
                      n204 = flat-sequence {
                        tunnel: [w709] -> w707
                        tunnel: w697 -> [w709]
                        frame #0 {
                          n205 = Wait (ms)(milliseconds to wait=u32 50) -> ()  [unwired: 1 out]
                        }
                      }
                      n206 = case shown="\"Velocity\"" w698 {
                        tunnel: [w713 w720 w730 w739 w758 "EP=1\r\n" ("write buffer") "Cannot perform operation.\n" ("read buffer")] -> w699
                        tunnel: w707 -> [w712 w719 w729 w744 w749 w761 w763]
                        tunnel: [w712 w719 w729 w744 w746 w761 w763] -> w706
                        tunnel: w704 -> [w714 w721 w735 _ _ _ _]
                        tunnel: w703 -> [_ _ _ w740 _ _ _]
                        tunnel: w702 -> [_ _ _ _ w750 _ _]
                        tunnel: w701 -> [_ w722 w733 _ _ _ _]
                        tunnel: "EP=1\r\n" ("string") -> [w711 w718 w728 w738 w745 _ _]
                        frame "Serial Number" {
                          n207 = Concatenate Strings(w711, "SN" ("write buffer"), "=" ("string"), w714, "\r\n" ("write buffer")) -> (w713:string)
                        }
                        frame "Temperature" {
                          n208 = Concatenate Strings(w718, "TA" ("string"), "[", w722, "]", "=" ("string"), w721, "\r\n" ("write buffer")) -> (w720:string)
                        }
                        frame "Unit Adress" {
                          n209 = Concatenate Strings(w728, "UA" ("string"), "[", w733, "]", "=" ("string"), w735, "\r\n" ("write buffer")) -> (w730:string)
                        }
                        frame "Calibration" {
                          n210 = Concatenate Strings(w738, "CC" ("string"), "=" ("string"), w740, "\r\n" ("write buffer")) -> (w739:string)
                        }
                        frame "Velocity" {
                          n211 = In Range and Coerce(upper limit=u16 18001, x=w750, lower limit=u16 0) -> (coerced(x)=w756:u32, In Range?=w754:bool)
                          n212 = Not(x=w754) -> (.not. x?=w755:bool)
                          n213 = Select(t=w756, s=w754, f=u16 0) -> (s? t:f=w748:u32)
                          n214 = Number To Decimal String(number=w748) -> (decimal integer string=w747:string)  [unwired: 1 in]
                          n215 = Concatenate Strings(w745, "VC" ("write buffer"), "=" ("string"), w747, "\r\n" ("write buffer")) -> (w758:string)
                          n216 = call "Display Message to User2"("error in (no error)"=w749, "Enable"=w755) -> ("error out"=w746:errorcluster)  [unwired: 8 in, 1 out]
                        }
                        frame "Enable Conf. EP=1" {
                        }
                        frame Default {
                        }
                      }
                      n217 = property on="read buffer" class="Str"() -> ("Value"=w696:string)  [unwired: 2 in, 2 out]
                      n218 = VISA Write(VISA resource name=w705, write buffer=w699, error in (no error)=w706) -> (error out=w708:errorcluster)  [unwired: 2 out]
                      n219 = Concatenate Strings(w696, w699) -> (w700:string)
                      n220 = property on="Serial Send" class="Bool (strict)"("Value"=w694) -> ()  [unwired: 2 in, 2 out]
                      n221 = flat-sequence {
                        tunnel: w708 -> [w765]
                        tunnel: [w765] -> w693
                        frame #0 {
                          n222 = Wait (ms)(milliseconds to wait=u32 50) -> ()  [unwired: 1 out]
                        }
                      }
                      n223 = property on="Get" class="Bool (strict)"(error in=w693, "Val(Sgnl)"=w691, "Value"=w691) -> (error out=w692:errorcluster)  [unwired: 1 in, 1 out]
                      n224 = property on="Set" class="Bool (strict)"("Value"=w694) -> ()  [unwired: 2 in, 2 out]
                    }
                  }
                }
              }
              "read buffer" <- w496
              n225 = Add(x=u32 5, y=w489) -> (x+y=w488:u32)
              n226 = property on="read buffer" class="Str"(error in=w491, "Text.Scroll Position"=w488) -> (error out=w490:errorcluster)  [unwired: 1 in, 1 out]
            }
            event "Set Param.": Value Change {
              n227 = event-data() -> ()  [unwired: 1 in, 6 out]
              n228 = property on="Serial Status" class="Bool (strict)"(error in=w771) -> (error out=w770:errorcluster, "Value"=w775:bool)  [unwired: 1 in, 1 out]
              n229 = case shown="True" w775 {
                tunnel: w770 -> [w787 w800]
                tunnel: [w786 w796] -> w773
                frame False {
                  n230 = call "Display Message to User4"("error in (no error)"=w787) -> ("error out"=w786:errorcluster)  [unwired: 9 in, 1 out]
                }
                frame True {
                  w789 = FALSE ("Visible")
                  n231 = property on="Speed control" class="Bool (strict)"(error in=w800, "Visible"=FALSE) -> (error out=w799:errorcluster)  [unwired: 1 in, 1 out]
                  n232 = case shown="47" "Param to Set" {
                    tunnel: [w853 w857 w861] -> w815
                    tunnel: w799 -> [w852 w856 w860]
                    tunnel: [w852 w856 w860] -> w803
                    frame 95, Default {
                      n233 = call <vilib>:"Application Directory.vi"() -> ("Application Directory"=w855:path)
                      n234 = Build Path(base path=w855, name or relative path="data\\Marvin_EBAY_params_RRPAR000017_95_v0.2.txt") -> (appended path=w853:path)
                    }
                    frame 63 {
                      n235 = call <vilib>:"Application Directory.vi"() -> ("Application Directory"=w859:path)
                      n236 = Build Path(base path=w859, name or relative path="data\\Marvin_AHU_params_RRPAR000016_63_v0.2.txt") -> (appended path=w857:path)
                    }
                    frame 47 {
                      n237 = call <vilib>:"Application Directory.vi"() -> ("Application Directory"=w863:path)
                      n238 = Build Path(base path=w863, name or relative path="data\\Marvin_AHU_params_RRPAR000015_47_v0.2.txt") -> (appended path=w861:path)
                    }
                  }
                  n239 = property on="read buffer" class="Str"(error in=w803, "Visible"=TRUE) -> (error out=w791:errorcluster)  [unwired: 1 in, 1 out]
                  n240 = property on="CAN Data" class="Arr (strict)"(error in=w791, "Visible"=w789) -> (error out=w790:errorcluster)  [unwired: 1 in, 1 out]
                  n241 = property on="PlayPause Data Array" class="Bool (strict)"("Visible"=w789) -> ()  [unwired: 2 in, 2 out]
                  n242 = property on="Clear Data Array" class="Bool (strict)"("Visible"=w789) -> ()  [unwired: 2 in, 2 out]
                  n243 = property on="Horizontal Progress Bar" class="Slide (strict)"(error in=w790, "Visible"=TRUE, "Value"=u8 0 ("Horizontal Progress Bar")) -> (error out=w798:errorcluster)  [unwired: 1 in, 1 out]
                  n244 = call <vilib>:"Read Characters From File.vi"("file path (dialog if empty)"=w815) -> ("character string"=w816:string)  [unwired: 5 in, 3 out]
                  n245 = while {
                    shift-right: [w844] -> _
                    shift-left: w816 -> [w845]
                    shift-right: [w840] -> w801
                    shift-left: string[] [] -> [w841]
                    tunnel: w798 -> [w833]
                    tunnel: [w833] -> w813
                    stop <- w846 stop-if-true
                    n246 = Match Pattern(string=w845, regular expression="\r\n") -> (before substring=w842:string, after substring=w844:string, offset past match=w843:i32)  [unwired: 1 in, 1 out]
                    n247 = call <vilib>:"Trim Whitespace.vi"("string"=w842) -> ("trimmed string"=w839:string)  [unwired: 1 in]
                    n248 = Equal?(x=w843, y=-1) -> (x = y?=w846:bool)
                    n249 = To Upper Case(1:w839) -> (0:w837:string)
                    n250 = String Length(string=w837) -> (length=w836:i32)
                    n251 = Greater?(x=w836, y=3) -> (0:w834:bool)
                    n252 = case shown="True" w834 {
                      tunnel: w841 -> [w848 w851]
                      tunnel: [w848 w850] -> w840
                      tunnel: w837 -> [_ w849]
                      frame False {
                      }
                      frame True {
                        n253 = Build Array (concatenate)(w851, w849) -> (w850:string[])
                      }
                    }
                  }
                  n254 = property on="VISA resource name" class="VISAName"(error in=w813) -> (error out=w806:errorcluster, "Value"=w795:refnum<visa-resource-name>)  [unwired: 1 in, 1 out]
                  n255 = Build Array (concatenate)(w801, string[] ["MT", "VR", "SN"] ("array")) -> (w810:string[])
                  n256 = Array Size(array=w810) -> (size(s)=w802:i32)
                  n257 = Bundle By Name(cluster=T12 {"Minimum"=0.0, "Maximum"=0.0, "Increment"=0.0} ("Data Entry Limits"), "Minimum"=0.0, "Maximum"=w802) -> (w808:T12)
                  n258 = property on="Horizontal Progress Bar" class="Slide (strict)"(error in=w806, "Data Range"=w808) -> (error out=w794:errorcluster)  [unwired: 1 in, 1 out]
                  n259 = property on="read buffer" class="Str"(error in=w794) -> (error out=w793:errorcluster, "Text.Scroll Position"=w792:u32)  [unwired: 1 in, 1 out]
                  n260 = for {
                    tunnel: w810 -> [w824] mode=indexing
                    tunnel: w795 -> [w830]
                    tunnel: w793 -> [w829]
                    tunnel: [w821] -> w797
                    tunnel: w792 -> [w820]
                    i -> [w819]
                    n261 = Concatenate Strings(w824, "\r\n" ("string")) -> (w822:string)
                    n262 = VISA Write(VISA resource name=w830, write buffer=w822, error in (no error)=w829) -> (error out=w828:errorcluster)  [unwired: 2 out]
                    n263 = flat-sequence {
                      tunnel: w828 -> [w831]
                      tunnel: [w831] -> w821
                      frame #0 {
                        n264 = Wait (ms)(milliseconds to wait=u32 50) -> ()  [unwired: 1 out]
                      }
                    }
                    n265 = Add(x=w820, y=w819) -> (x+y=w818:u32)
                    n266 = feedback #1("") -> (w826:string)
                    n267 = Concatenate Strings(w826, w822) -> (w827:string)
                    n268 = feedback-in #1(w827) -> ()
                    n269 = property on="read buffer" class="Str"("Value"=w827, "Text.Scroll Position"=w818) -> ()  [unwired: 2 in, 2 out]
                    "Horizontal Progress Bar" <- w819
                  }
                  n270 = VISA Flush I/O Buffer(VISA resource name=w795, error in (no error)=w797) -> (error out=w796:errorcluster)  [unwired: 1 in, 1 out]
                }
              }
              n271 = property on="Serial Monitor" class="Bool (strict)"(error in=w773) -> (error out=w772:errorcluster, "Value"=w774:bool)  [unwired: 1 in, 1 out]
              n272 = case shown="False" w774 {
                tunnel: w772 -> [w784 w785]
                tunnel: [w781 w785] -> w768
                frame False {
                  w780 = TRUE ("Visible")
                  n273 = property on="PlayPause Data Array" class="Bool (strict)"("Visible"=w780) -> ()  [unwired: 2 in, 2 out]
                  n274 = property on="read buffer" class="Str"(error in=w784, "Visible"=FALSE) -> (error out=w782:errorcluster)  [unwired: 1 in, 1 out]
                  n275 = property on="Clear Data Array" class="Bool (strict)"("Visible"=w780) -> ()  [unwired: 2 in, 2 out]
                  n276 = property on="CAN Data" class="Arr (strict)"(error in=w782, "Visible"=w780) -> (error out=w781:errorcluster)  [unwired: 1 in, 1 out]
                }
                frame True {
                }
              }
              n277 = call "Display Message to User5"("error in (no error)"=w768) -> ("error out"=w767:errorcluster)  [unwired: 9 in, 1 out]
            }
            event "Help Button": Value Change {
              n278 = event-data() -> ()  [unwired: 1 in, 6 out]
              n279 = control-ref of="This VI"() -> (w872:refnum<vi>)
              n280 = property class="VI"(reference=w872, error in=w870, "FP:Transparency"=u8 25 ("Front Panel Window:Transparency")) -> (reference out=w866:refnum<vi>, error out=w869:errorcluster)
              n281 = vi-ref "Help.vi"() -> (w876:refnum<vi>)
              n282 = invoke class="VI" method="FP.Open"(reference=w876, error in=w869, "Activate"=TRUE ("Activate?"), "State"=T13."Standard") -> (error out=w875:errorcluster)  [unwired: 1 in, 4 out]
              n283 = call "Help.vi"("error in"=w875, "TesterSWVersion"="1.7") -> ("error out"=w868:errorcluster)  [unwired: 6 in]
              n284 = property class="VI"(reference=w866, error in=w868, "FP:Transparency"=u8 0 ("Front Panel Window:Transparency")) -> (error out=w867:errorcluster)  [unwired: 1 out]
            }
            event "Can Send": Value Change {
              w904 = u8 0 items=["STATUS"=128, "EXTENDED"=2, "RTR"=1, "DATA MSG"=0] ("MSGTYPE")
              w909 = u8 1 items=["Standart flag", "Extern flag"] ("Format")
              w908 = u8 0 items=["Data flag", "Remote flag"] ("Type")
              # "Send"
              n285 = event-data() -> ()  [unwired: 1 in, 6 out]
              n286 = disable-structure shown="Disabled" {
                disable-tunnel: "Motor Phase Current" -> [w922 _]
                frame Disabled {
                  w923 = u16 40 ("lower limit")
                  n287 = In Range and Coerce(upper limit=u16 100, x=w922, lower limit=w923) -> (coerced(x)=w925:u16, In Range?=w927:bool)
                  n288 = Not(x=w927) -> (.not. x?=w926:bool)
                  n289 = call "Display Message to User6"("Enable"=w926) -> ()  [unwired: 9 in, 2 out]
                  n290 = Select(t=w925, s=w927, f=w923) -> ()  [unwired: 1 out]
                }
                frame Enabled {
                }
              }
              n291 = In Range and Coerce(upper limit=u16 18001, x="Motor Speed RPM", lower limit=u16 0) -> (coerced(x)=w891:u16, In Range?=w889:bool)
              n292 = Not(x=w889) -> (.not. x?=w890:bool)
              n293 = call "Display Message to User"("Enable"=w890) -> ()  [unwired: 9 in, 2 out]
              n294 = Select(t=w891, s=w889, f=u16 0) -> (s? t:f=w893:u16)
              n295 = property on="UUT" class="DigNum (strict)"() -> ("Value"=w887:u8)  [unwired: 2 in, 2 out]
              n296 = Split Number(x=w893) -> (hi(x)=w896:u8, lo(x)=w897:u8)
              n297 = case shown="79" w887 {
                tunnel: [u32 417357607 u32 417353511 u32 417349415 u32 417345319] -> w888
                frame 95, Default {
                }
                frame 79 {
                }
                frame 63 {
                }
                frame 47 {
                }
              }
              n298 = case shown="79" w887 {
                tunnel: [w934 w943 w956 w970] -> w902
                tunnel: w897 -> [w933 w942 w955 w969]
                tunnel: w896 -> [w932 w941 w954 w968]
                tunnel: "Motor Speed RPM" -> [w929 w938 _ _]
                tunnel: "Speed control" -> [_ _ w947 w961]
                tunnel: "Motor Over Temp" -> [_ _ w946 w960]
                tunnel: "Motor Phase Current" -> [_ _ _ w957]
                frame 47, Default {
                  w931 = u8 0 ("element")
                  n299 = case shown="1, Default" w929 {
                    tunnel: [u8 1 ("element") u8 0 ("element")] -> w928
                    frame 1, Default {
                    }
                    frame 0 {
                    }
                  }
                  n300 = Build Array(u8 1 ("element"), w933, w932, w928, w931, w931, w931, w931) -> (w934:u8[])
                }
                frame 63 {
                  w939 = u8 0 ("element")
                  n301 = case shown="1, Default" w938 {
                    tunnel: [u8 1 ("element") u8 0 ("element")] -> w937
                    frame 1, Default {
                    }
                    frame 0 {
                    }
                  }
                  n302 = Build Array(u8 1 ("element"), w942, w941, w937, w939, w939, w939, w939) -> (w943:u8[])
                }
                frame 95 {
                  w952 = u8 0 ("element")
                  n303 = Boolean To (0,1)(Boolean=w947) -> (0, 1=w950:i16)
                  n304 = Boolean To (0,1)(Boolean=w946) -> (0, 1=w951:i16)
                  n305 = To Unsigned Byte Integer(number=w950) -> (unsigned 8bit integer=w949:u8)
                  n306 = To Unsigned Byte Integer(number=w951) -> (unsigned 8bit integer=w948:u8)
                  n307 = Build Array(u8 1 ("element"), w955, w954, w949, w948, w952, w952, w952) -> (w956:u8[])
                }
                frame 79 {
                  n308 = Split Number(x=w957) -> (hi(x)=w958:u8, lo(x)=w959:u8)
                  n309 = Boolean To (0,1)(Boolean=w961) -> (0, 1=w964:i16)
                  n310 = Boolean To (0,1)(Boolean=w960) -> (0, 1=w965:i16)
                  n311 = To Unsigned Byte Integer(number=w964) -> (unsigned 8bit integer=w963:u8)
                  n312 = To Unsigned Byte Integer(number=w965) -> (unsigned 8bit integer=w962:u8)
                  n313 = Build Array(u8 1 ("element"), w969, w968, w963, w962, w959, w958, u8 0 ("element")) -> (w970:u8[])
                }
              }
              n314 = Array Size(array=w902) -> (size(s)=w907:i32)
              n315 = call "Array Data to Single Num in Hex.vi"("aDATA"=w902) -> ("Numeric"=→"Data Send":u64)  [unwired: 10 in]
              n316 = To Unsigned Byte Integer(number=w907) -> (unsigned 8bit integer=w905:u8)
              n317 = call "CANAnalData.vi"("ID"=w888, "Data"=w902, "Config"=w900) -> ()  [unwired: 4 in, 5 out]
              n318 = Bundle By Name(cluster=T10 {"ID"=0, "MSGTYPE"=0, "LEN"=0, "aDATA"=[]} ("MsgTX 2"), "ID"=w888, "MSGTYPE"=w904, "LEN"=w905, "aDATA"=w902) -> (w903:T10)
              n319 = Unbundle By Name(w903) -> ("ID"=w917:u32, "LEN"=w918:u8, "aDATA"=w919:u8[])  [unwired: 1 out]
              n320 = property class="Clust (strict)"(reference=w900) -> ("Value"=w916:T8)  [unwired: 1 in, 2 out]
              n321 = Bundle By Name(cluster=T14 {"ID"=0, "TimeStamp"=0, "TimeFlag"=0, "SendType"=0, "RemoteFlag"=0, "ExternFlag"=0, "DataLen"=0, "Data"=[], "Reserved"=[]} ("Send"), "ID"=w917, "RemoteFlag"=w908, "ExternFlag"=w909, "DataLen"=w918, "Data"=w919) -> (w914:T14)
              n322 = Unbundle By Name(w916) -> ("DevType"=w910:T2, "DevIndex"=w911:u32, "CanIndex"=w912:T3)
              n323 = Build Array(w914) -> (w913:T14[])
              n324 = call "VCI_Transmit.vi"("Buffer"=w913, "CANIndex"=w912, "DevIndex"=w911, "DevType"=w910) -> ()  [unwired: 1 in, 7 out]
            }
            event "Graph Button": Value Change {
              w976 = FALSE ("Visible")
              w978 = FALSE ("Visible")
              n325 = event-data() -> ()  [unwired: 1 in, 6 out]
              n326 = Not(x="Graph Button") -> (.not. x?=w979:bool)
              n327 = property on="PlayPause Data Array" class="Bool (strict)"("Visible"=w979) -> ()  [unwired: 2 in, 2 out]
              n328 = property on="CAN Data" class="Arr (strict)"(error in=w980, "Visible"=w979) -> (error out=w981:errorcluster)  [unwired: 1 in, 1 out]
              n329 = property on="Clear Data Array" class="Bool (strict)"("Visible"=w979) -> ()  [unwired: 2 in, 2 out]
              n330 = property on="Waveform Chart" class="WFChart (strict)"(error in=w981, "Visible"="Graph Button") -> (error out=w983:errorcluster)  [unwired: 1 in, 1 out]
              n331 = property on="Serial Monitor" class="Bool (strict)"(error in=w983) -> (error out=w996:errorcluster, "Value"=w997:bool)  [unwired: 1 in, 1 out]
              n332 = case shown="True" w997 {
                tunnel: w996 -> [w1004 w1009]
                tunnel: [w1002 w1006] -> w986
                frame False {
                  n333 = property on="read buffer" class="Str"(error in=w1004, "Visible"=FALSE) -> (error out=w1002:errorcluster)  [unwired: 1 in, 1 out]
                }
                frame True {
                  w1005 = FALSE ("Visible")
                  n334 = property on="PlayPause Data Array" class="Bool (strict)"("Visible"=w1005) -> ()  [unwired: 2 in, 2 out]
                  n335 = property on="read buffer" class="Str"(error in=w1009, "Visible"=TRUE) -> (error out=w1007:errorcluster)  [unwired: 1 in, 1 out]
                  n336 = property on="Clear Data Array" class="Bool (strict)"("Visible"=w1005) -> ()  [unwired: 2 in, 2 out]
                  n337 = property on="CAN Data" class="Arr (strict)"(error in=w1007, "Visible"=w1005) -> (error out=w1006:errorcluster)  [unwired: 1 in, 1 out]
                }
              }
              n338 = property on="Serial Monitor" class="Bool (strict)"(error in=w986, "Value"=FALSE ("Serial Monitor")) -> (error out=w984:errorcluster)  [unwired: 1 in, 1 out]
              n339 = property on="Index" class="Ring (strict)"(error in=w984, "Visible"=w978) -> (error out=w993:errorcluster)  [unwired: 1 in, 1 out]
              n340 = property on="Value 1/2" class="Enum (strict)"(error in=w993, "Visible"=w978) -> (error out=w992:errorcluster)  [unwired: 1 in, 1 out]
              n341 = property on="Value" class="DigNum (strict)"(error in=w992, "Visible"=w978) -> (error out=w991:errorcluster)  [unwired: 1 in, 1 out]
              n342 = property on="SetGet" class="Enum (strict)"(error in=w991, "Visible"=w978) -> (error out=w975:errorcluster)  [unwired: 1 in, 1 out]
              n343 = property on="Set" class="Bool (strict)"(error in=w975, "Visible"=w976) -> (error out=w977:errorcluster)  [unwired: 1 in, 1 out]
              n344 = property on="Get" class="Bool (strict)"(error in=w977, "Visible"=w976) -> ()  [unwired: 1 in, 2 out]
              n345 = property on="Serial Send" class="Bool (strict)"(error in=w975, "Visible"=w978) -> (error out=w989:errorcluster)  [unwired: 1 in, 1 out]
              n346 = property on="Clear Monitor" class="Bool"(error in=w989, "Visible"=w978) -> (error out=w988:errorcluster)  [unwired: 1 in, 1 out]
              n347 = property on="Function" class="Enum (strict)"(error in=w988, "Visible"=w978) -> (error out=w990:errorcluster)  [unwired: 1 in, 1 out]
              n348 = property on="Index" class="Ring (strict)"(error in=w990, "Visible"=w978) -> (error out=w994:errorcluster)  [unwired: 1 in, 1 out]
              n349 = property on="read buffer" class="Str"(error in=w994, "Visible"=w978) -> (error out=w987:errorcluster)  [unwired: 1 in, 1 out]
            }
            event "Serial Com": Value Change {
              n350 = event-data() -> ()  [unwired: 1 in, 6 out]
              n351 = property on="Serial Com" class="Bool"(error in=w1014, "Visible"=FALSE) -> (error out=w1013:errorcluster)  [unwired: 1 in, 1 out]
              n352 = property on="VISA resource name" class="VISAName"(error in=w1013, "Visible"=TRUE) -> (error out=w1011:errorcluster)  [unwired: 1 in, 1 out]
            }
            event "VISA resource name": Value Change {
              n353 = event-data() -> ()  [unwired: 1 in, 1 out]
              n354 = control-ref of="This VI"() -> (w1020:refnum<vi>)
              n355 = call "Serial InitMarvin.vi"("error in (no error)"=w1029, "VI reference (current VI)"=w1020, "VISA Refnum in"="VISA resource name") -> ("error out"=w1038:errorcluster, "Boolean"=w1026:bool)  [unwired: 7 in]
              n356 = property on="Serial Status" class="Bool (strict)"(error in=w1038, "Value"=w1026) -> (error out=w1032:errorcluster)  [unwired: 1 in, 1 out]
              n357 = property on="VISA resource name" class="VISAName"(error in=w1032, "Visible"=FALSE) -> (error out=w1031:errorcluster)  [unwired: 1 in, 1 out]
              n358 = property on="Serial Com" class="Bool"(error in=w1031, "Visible"=TRUE) -> (error out=w1024:errorcluster)  [unwired: 1 in, 1 out]
              n359 = call "Serial.vi"("error in (no error)"=w1024, "Clear Log"=TRUE, "VISA resource name"="VISA resource name") -> ("error out"=w1022:errorcluster)  [unwired: 7 in, 1 out]
              n360 = call <vilib>:"Clear Errors.vi"("error in (no error)"=w1022) -> ("error out"=w1028:errorcluster)  [unwired: 5 in, 1 out]
              n361 = case shown="True" w1026 {
                tunnel: w1028 -> [w1039 w1042]
                tunnel: [w1039 w1041] -> w1027
                tunnel: "VISA resource name" -> [_ w1040]
                frame False {
                }
                frame True {
                  n362 = VISA Flush I/O Buffer(VISA resource name=w1040, error in (no error)=w1042) -> (error out=w1041:errorcluster)  [unwired: 1 in, 1 out]
                }
              }
            }
            event "Stop": Value Change {
              n363 = event-data() -> ()  [unwired: 1 in, 6 out]
              n364 = Flush Queue(queue=w1048, error in (no error)=w1047) -> (queue out=w1046:refnum<queue>, error out=w1045:errorcluster)  [unwired: 1 out]
              n365 = Release Queue(queue=w1046, error in (no error)=w1045) -> (error out=w1044:errorcluster)  [unwired: 1 in, 2 out]
            }
            event "Refresh Button", "Graph Plot": Value Change {
              n366 = event-data() -> ("CtlRef"=w1055:refnum<vi>)  [unwired: 1 in, 5 out]
              n367 = property class="Bool"(reference=w1055) -> ("Label.Text"=w1054:string)  [unwired: 1 in, 2 out]
              n368 = case shown="\"Graph Plot\"" w1054 {
                tunnel: w1059 -> [w1064 w1068 w1073]
                tunnel: w1058 -> [_ _ w1072]
                tunnel: [w1065 w1068 w1071] -> w1057
                tunnel: [FALSE ("Stop") FALSE ("Stop") TRUE ("Stop")] -> w1053
                tunnel: [enum16{"Stop", "MainProgram", "Initialize"}."MainProgram" enum16{"Stop", "MainProgram", "Initialize"}."MainProgram" enum16{"Stop", "MainProgram", "Initialize"}."Initialize"] -> w1052
                frame "Graph Plot" {
                  n369 = property on="Waveform Chart" class="WFChart (strict)"(error in=w1064, "History Data"=dbl[] [] ("Waveform Chart")) -> (error out=w1065:errorcluster)  [unwired: 1 in, 1 out]
                }
                frame Default {
                }
                frame "Refresh Button" {
                  n370 = Release Queue(queue=w1072, error in (no error)=w1073) -> (error out=w1071:errorcluster)  [unwired: 1 in, 2 out]
                }
              }
            }
          }
          n371 = Unbundle By Name(w283) -> ("status"=w289:bool)
          n372 = Or(x=w289, y=w281) -> (x .or. y?=w288:bool)
        }
        n373 = while {
          shift-right: [w124] -> _
          shift-left: w101 -> [w125]
          shift-right: [w122] -> _
          shift-left: _ -> [w123]
          shift-right: [w118] -> _
          shift-left: w100 -> [w118]
          shift-right: [w107] -> w96
          shift-left: w97 -> [w110]
          shift-right: [w111] -> _
          shift-left: cluster{"Frame Data":u64, "Frame ID":u32}[] [] ("Array 3") -> [w113]
          stop <- w108 stop-if-true
          n374 = Dequeue Element(queue=w125, error in (no error)=w118) -> (queue out=w124:refnum<queue>, element=w119:T9, error out=w108:errorcluster)  [unwired: 1 in, 1 out]
          n375 = for {
            tunnel: [w267] -> w121 mode=indexing
            tunnel: w119 -> [w269] mode=indexing
            tunnel: [w268] -> w120 mode=indexing
            tunnel: [w266] -> w117 mode=indexing
            tunnel: [w265] -> w116 mode=indexing
            shift-right: [w265] -> _
            shift-left: _ -> [w264]
            n376 = Unbundle By Name(w269) -> ("ID"=w266:u32, "aDATA"=w268:u8[])
            n377 = call "Array Data to Single Num in Hex.vi"("aDATA"=w268) -> ("Numeric"=w267:u64)  [unwired: 10 in]
            n378 = case shown="Default" w266 {
              tunnel: w267 -> [_ w274]
              tunnel: w266 -> [_ w273]
              tunnel: [w270 w272] -> w265
              tunnel: w264 -> [w270 _]
              frame 0 {
              }
              frame Default {
                n379 = Bundle By Name(cluster=cluster{"Frame Data":u64, "Frame ID":u32} {"Frame Data"=0, "Frame ID"=0} ("Cluster"), "Frame ID"=w273, "Frame Data"=w274) -> (w272:cluster{"Frame Data":u64, "Frame ID":u32})
              }
            }
          }
          n380 = case shown="True" "PlayPause Data Array" {
            tunnel: w116 -> [w128 _]
            tunnel: w113 -> [w127 w129]
            tunnel: [w126 w129] -> w112
            frame False {
              n381 = Build Array (concatenate)(w128, w127) -> (w126:cluster{"Frame Data":u64, "Frame ID":u32}[])
            }
            frame True {
            }
          }
          n382 = Build Array (concatenate)(w121, w123) -> (w122:u64[][])
          "Array" <- w122
          n383 = Select(t=cluster{"Frame Data":u64, "Frame ID":u32}[] [], s="Clear Data Array", f=w112) -> (s? t:f=w111:cluster{"Frame Data":u64, "Frame ID":u32}[])
          "CAN Data" <- w111
          n384 = for {
            tunnel: w120 -> [w133] mode=indexing
            tunnel: w117 -> [w131] mode=indexing
            shift-right: [w130] -> w107
            shift-left: w110 -> [w132]
            n385 = case shown="417474351, 417474367, 417474383, 417474399" w131 {
              tunnel: w133 -> [_ w163 w201 w259]
              tunnel: [w134 w136 w192 w231] -> w130
              tunnel: w132 -> [w134 w140 w192 w232]
              frame Default {
              }
              frame 417408815, 417408831, 417408847, 417408863 {
                # "Frame ID\n0x18E1273F"
                n386 = Index Array(array=w163, index #1=0 ("index"), index #2=1 ("index"), index #3=2 ("index"), index #4=3 ("index"), index #5=4 ("index"), index #6=5 ("index"), index #7=6 ("index"), index #8=7 ("index")) -> (element #1=w147:u8, element #2=w149:u8, element #3=w150:u8, element #4=w154:u8, element #5=w157:u8, element #6=w161:u8, element #7=w162:u8, element #8=w160:u8)
                n387 = Join Numbers(hi=w162, lo=w161) -> ((hi.lo)=w181:u16)
                n388 = Join Numbers(hi=w150, lo=w149) -> ((hi.lo)=w151:u16)
                n389 = Number To Hexadecimal String(2:w181) -> (0:w180:string)  [unwired: 1 in]
                n390 = Number To Hexadecimal String(2:w160) -> (0:w174:string)  [unwired: 1 in]
                n391 = Number To Hexadecimal String(2:w147) -> (0:w148:string)  [unwired: 1 in]
                n392 = Number To Hexadecimal String(2:w151) -> (0:w152:string)  [unwired: 1 in]
                n393 = Number To Hexadecimal String(2:w154) -> (0:w155:string)  [unwired: 1 in]
                n394 = Number To Hexadecimal String(2:w157) -> (0:w158:string)  [unwired: 1 in]
                n395 = Hexadecimal String To Number(string=w148) -> (number=w145:u32)  [unwired: 2 in, 1 out]
                n396 = Hexadecimal String To Number(string=w152) -> (number=w153:u32)  [unwired: 2 in, 1 out]
                n397 = Hexadecimal String To Number(string=w155) -> (number=w156:u32)  [unwired: 2 in, 1 out]
                n398 = Hexadecimal String To Number(string=w158) -> (number=w159:u32)  [unwired: 2 in, 1 out]
                n399 = Hexadecimal String To Number(string=w174) -> (number=w173:u32)  [unwired: 2 in, 1 out]
                n400 = Hexadecimal String To Number(string=w180) -> (number=w179:u32)  [unwired: 2 in, 1 out]
                n401 = To Unsigned Word Integer(number=w145) -> (unsigned 16bit integer=→"ECS State":u16)
                n402 = To Double Precision Float(number=w153) -> (double precision float=w139:dbl)
                "Motor Speed RPM" <- w139
                n403 = To Double Precision Float(number=w179) -> (double precision float=w176:dbl)
                n404 = To Double Precision Float(number=w173) -> (double precision float=→"Phase Current":dbl)
                n405 = To Double Precision Float(number=w156) -> (double precision float=w144:dbl)
                n406 = To Double Precision Float(number=w159) -> (double precision float=w142:dbl)
                n407 = To Double Precision Float(number=u32 10 ("y")) -> (double precision float=w177:dbl)
                n408 = Subtract(x=w142, y=50.0 ("x")) -> (x-y=→"Power transistor Heat sink Temp.":dbl)
                n409 = Subtract(x=w144, y=50.0 ("x")) -> (x-y=→"Motor Stator Temp.":dbl)
                n410 = Divide(x=w176, y=w177) -> (x/y=→"DC Voltage":dbl)
                n411 = case shown="False" "Graph Plot" {
                  tunnel: w140 -> [w184 w189]
                  tunnel: [w182 w189] -> w136
                  tunnel: w139 -> [w183 _]
                  frame False {
                    n412 = disable-structure shown="Disabled" {
                      disable-tunnel: w183 -> [w188 _]
                      frame Disabled {
                        n413 = call <vilib>:"Application Directory.vi"() -> ("Application Directory"=w186:path)
                        n414 = Build Path(base path=w186, name or relative path="RPM Log.lvm") -> (appended path=w187:path)
                        n415 = call "Write To Measurement File"("Signals"=w188, "Filename"=w187) -> ()  [unwired: 15 in, 3 out]
                      }
                      frame Enabled {
                      }
                    }
                    n416 = Build Array (concatenate)(w183, w184) -> (w182:dbl[])
                    "Waveform Chart" <- w183
                  }
                  frame True {
                  }
                }
              }
              frame 417539887, 417539903, 417539919, 417539935 {
                # "Framde ID\n0x18E3273F"
                n417 = property on="UUT" class="DigNum (strict)"() -> ("Value"=w191:u8)  [unwired: 2 in, 2 out]
                n418 = Index Array(array=w201, index #1=0 ("index"), index #2=1 ("index")) -> (element #1=w199:u8, element #2=w194:u8)
                n419 = case shown="Default" w191 {
                  tunnel: [0 1 2] -> w190
                  frame Default {
                  }
                  frame 95 {
                  }
                  frame 79 {
                  }
                }
                n420 = Number To Boolean Array(number=w199) -> (Boolean array=w198:bool[])
                n421 = Number To Boolean Array(number=w194) -> (Boolean array=w196:bool[])
                n422 = Boolean To (0,1)(Boolean=w196) -> (0, 1=w193:i16[])
                n423 = Boolean To (0,1)(Boolean=w198) -> (0, 1=w197:i16[])
                n424 = case shown="79, 95" w191 {
                  tunnel: w193 -> [_ w206]
                  tunnel: w190 -> [_ w205]
                  frame 0, Default {
                  }
                  frame 79, 95 {
                    n425 = for {
                      tunnel: w206 -> [w211] mode=indexing
                      tunnel: w205 -> [w207]
                      i -> [w208]
                      stop <- w209 stop-if-true
                      n426 = Not Equal To 0?(x=w211) -> (x != 0?=w210:bool)
                      n427 = case shown="2" w208 {
                        tunnel: w210 -> [w212 w213 w214]
                        frame 0, Default {
                          "Ambient Sensor temp" <- w212
                        }
                        frame 1 {
                          "Ambient Over temp" <- w213
                        }
                        frame 2 {
                          "Hall Sensor Fault" <- w214
                        }
                      }
                      n428 = Equal?(x=w208, y=w207) -> (x = y?=w209:bool)
                    }
                  }
                }
                n429 = for {
                  tunnel: w197 -> [w216] mode=indexing
                  i -> [w217]
                  n430 = Not Equal To 0?(x=w216) -> (x != 0?=w215:bool)
                  n431 = case shown="0, Default" w217 {
                    tunnel: w215 -> [w218 w219 w220 w221 w222 w223 w224 w225]
                    frame 0, Default {
                      "Drive Sensor temp Failure" <- w218
                    }
                    frame 1 {
                      "Drive Over temperature" <- w219
                    }
                    frame 2 {
                      "Motor Sensor temp Fauilre" <- w220
                    }
                    frame 3 {
                      "Motor Over temperature" <- w221
                    }
                    frame 4 {
                      "Derated drive temp" <- w222
                    }
                    frame 5 {
                      "Under voltage/Over voltage" <- w223
                    }
                    frame 6 {
                      "Commutation err" <- w224
                    }
                    frame 7 {
                      "Speed error" <- w225
                    }
                  }
                }
              }
              frame 417474351, 417474367, 417474383, 417474399 {
                w242 = "."
                # "Frame ID\n0x18E2273F"
                n432 = Index Array(array=w259, index #1=0 ("index")) -> (element #1=w257:u8, element #2=w255:u8, element #3=w236:u8, element #4=w237:u8, element #5=w238:u8, element #6=w239:u8)  [unwired: 5 in]
                n433 = Split Number(x=w238) -> (hi(x)=w250:u8, lo(x)=w249:u8)
                n434 = Split Number(x=w239) -> (hi(x)=w248:u8, lo(x)=w247:u8)
                n435 = Join Numbers(hi=w237, lo=w236) -> ((hi.lo)=w228:u16)
                n436 = Number To Hexadecimal String(2:w228) -> (0:w229:string)  [unwired: 1 in]
                n437 = Number To Decimal String(number=w250) -> (decimal integer string=w246:string)  [unwired: 1 in]
                n438 = Number To Decimal String(number=w249) -> (decimal integer string=w245:string)  [unwired: 1 in]
                n439 = Number To Decimal String(number=w248) -> (decimal integer string=w244:string)  [unwired: 1 in]
                n440 = Number To Decimal String(number=w247) -> (decimal integer string=w243:string)  [unwired: 1 in]
                n441 = Hexadecimal String To Number(string=w229) -> (number=w230:u32)  [unwired: 2 in, 1 out]
                n442 = To Double Precision Float(number=w230) -> (double precision float=w227:dbl)
                n443 = Number To Hexadecimal String(2:w255) -> (0:w253:string)  [unwired: 1 in]
                n444 = To Double Precision Float(number=w257) -> (double precision float=→"Motor Phase Current RMS":dbl)
                n445 = Multiply(x=w227, y=u16 1) -> (x*y=w234:dbl)
                n446 = Concatenate Strings(w246, w242, w245, w242, w244, w242, w243) -> (→"Driver Version":string)
                n447 = To Double Precision Float(number=w234) -> (double precision float=w233:dbl)
                "Motor Phase Current" <- w233
                n448 = Hexadecimal String To Number(string=w253) -> (number=w254:u32)  [unwired: 2 in, 1 out]
                n449 = To Double Precision Float(number=w254) -> (double precision float=w252:dbl)
                n450 = Subtract(x=w252, y=50.0) -> (x-y=→"Ambient Temperature":dbl)
                n451 = property on="Graph Plot" class="Bool (strict)"() -> ("Value"=w226:bool)  [unwired: 2 in, 2 out]
                n452 = case shown="True" w226 {
                  tunnel: w232 -> [w260 w263]
                  tunnel: [w260 w262] -> w231
                  tunnel: w233 -> [_ w261]
                  frame False {
                  }
                  frame True {
                    n453 = property on="Waveform Chart" class="WFChart (strict)"("Value"=w261) -> ()  [unwired: 2 in, 2 out]
                    n454 = Build Array (concatenate)(w261, w263) -> (w262:dbl[])
                  }
                }
              }
            }
            "Array 2" <- w130
          }
        }
      }
      frame "Stop" {
        n455 = Release Queue(queue=w1078, error in (no error)=w1080) -> (error out=w1079:errorcluster)  [unwired: 1 in, 2 out]
        n456 = flat-sequence {
          tunnel: w1077 -> [w1081]
          tunnel: [TRUE ("Stop")] -> w1076
          frame #0 {
            w1087 = u8[] [1, 0, 0, 0, 0, 0, 0, 0] ("Data 2")
            w1089 = u8 0 items=["STATUS"=128, "EXTENDED"=2, "RTR"=1, "DATA MSG"=0] ("MSGTYPE")
            w1094 = u8 1 items=["Standart flag", "Extern flag"] ("Format")
            w1093 = u8 0 items=["Data flag", "Remote flag"] ("Type")
            n457 = property on="Serial Status" class="Bool (strict)"() -> ("Value"=w1082:bool)  [unwired: 2 in, 2 out]
            n458 = property on="UUT" class="DigNum (strict)"() -> ("Value"=w1084:u8)  [unwired: 2 in, 2 out]
            n459 = case shown="True" w1082 {
              frame False {
              }
              frame True {
                n460 = property on="VISA resource name" class="VISAName"() -> ("Value"=w1105:refnum<visa-resource-name>)  [unwired: 2 in, 2 out]
                n461 = VISA Close(VISA resource name=w1105) -> ()  [unwired: 1 in, 1 out]
              }
            }
            n462 = case shown="95, Default" w1084 {
              tunnel: [u32 417357607 u32 417349415 u32 417345319] -> w1083
              frame 95, Default {
              }
              frame 63 {
              }
              frame 47 {
              }
            }
            n463 = property on="Graph Button" class="Bool (strict)"("Value"=FALSE ("Graph Button")) -> ()  [unwired: 2 in, 2 out]
            n464 = Array Size(array=w1087) -> (size(s)=w1092:i32)
            n465 = To Unsigned Byte Integer(number=w1092) -> (unsigned 8bit integer=w1090:u8)
            n466 = Bundle By Name(cluster=T10 {"ID"=0, "MSGTYPE"=0, "LEN"=0, "aDATA"=[]} ("MsgTX 2"), "ID"=w1083, "MSGTYPE"=w1089, "LEN"=w1090, "aDATA"=w1087) -> (w1088:T10)
            n467 = call "CANAnalData.vi"("ID"=w1083, "Data"=w1087, "Config"=w1081) -> ()  [unwired: 4 in, 5 out]
            n468 = call "Array Data to Single Num in Hex.vi"("aDATA"=w1087) -> ("Numeric"=w1086:u64)  [unwired: 10 in]
            n469 = property on="Data Send" class="DigNum (strict)"("Value"=w1086) -> ()  [unwired: 2 in, 2 out]
            n470 = Unbundle By Name(w1088) -> ("ID"=w1102:u32, "LEN"=w1103:u8, "aDATA"=w1104:u8[])  [unwired: 1 out]
            n471 = property class="Clust (strict)"(reference=w1081) -> ("Value"=w1101:T8)  [unwired: 1 in, 2 out]
            n472 = Bundle By Name(cluster=T14 {"ID"=0, "TimeStamp"=0, "TimeFlag"=0, "SendType"=0, "RemoteFlag"=0, "ExternFlag"=0, "DataLen"=0, "Data"=[], "Reserved"=[]} ("Send"), "ID"=w1102, "RemoteFlag"=w1093, "ExternFlag"=w1094, "DataLen"=w1103, "Data"=w1104) -> (w1099:T14)
            n473 = Unbundle By Name(w1101) -> ("DevType"=w1095:T2, "DevIndex"=w1096:u32, "CanIndex"=w1097:T3)
            n474 = Build Array(w1099) -> (w1098:T14[])
            n475 = call "VCI_Transmit.vi"("Buffer"=w1098, "CANIndex"=w1097, "DevIndex"=w1096, "DevType"=w1095) -> ()  [unwired: 1 in, 7 out]
          }
          frame #1 {
          }
        }
      }
    }
  }
  n476 = disable-structure shown="Disabled" {
    frame Disabled {
      n477 = control-ref of="Config_CANAT"() -> ()  [unwired: 1 out]
      n478 = control-ref of="UUT"() -> ()  [unwired: 1 out]
    }
    frame Enabled {
    }
  }
